vi "Edit_Maths_Equation.vi"(3 "Template Info Array":T1[](array[typedef]) {"Tolerance" min=0.0 format="%#.4f"}, 4 "Maths Equation In":string, 5 "Channel Name":string) -> (0 "Template Info Array Out":T1[](array[typedef]) {"Tolerance" min=0.0 format="%#.4f"}, 1 "Maths Equation Out":string)   [LabVIEW 2016]
uses:
  File_Template_Clus.ctl
  Data plotting/subVIs/Dispose_Channel.ctl
panel:
  in  "K 9":u16(ring) items=["File::", "Date::", "Time::", "Comments::", "Chilled Water:Temp:", "Inlet_Temp:Average:", "Av:Floor:Temp", "Max:deltaT:", "X (mm)::", "Y (mm)::", "Z (mm)::", "Z (m)::", "U/Uref::", "u^2/Uref^2::", "w^2/Uref^2::", "-uw/Uref^2::", "Inlet:DeltaT:", "DeltaT::", "t^2::", "ut::", "wt::", "Grad:Ri:", "Flux:Ri:", "B-V:Freq:N", "DeltaT/DeltaTmax::", "W/Uref::", "T:thermistor:", "dT/dZ::", "dU/dZ::", "Inlet:Delta_Set:", "u'/U::", "w'/U::", "W/U::", "Location:XY:", "Location:XZ:", "U:m/s:", "W:m/s:", "u^2::", "w^2::", "Speed/Uref::", "T:cw:", "Uref::", "Flow:Meas:Time", "Profile::", "t'/T::", "t'::", "uw::", "Spires::", "Roughness::", "Z=1450:Inlet:Temp", "Z=1350:Inlet:Temp", "Z=1250:Inlet:Temp", "Z=1150:Inlet:Temp", "Z=1050:Inlet:Temp", "Z=950:Inlet:Temp", "Z=850:Inlet:Temp", "Z=750:Inlet:Temp", "Z=650:Inlet:Temp", "Z=550:Inlet:Temp", "Z=450:Inlet:Temp", "Z=350:Inlet:Temp", "Z=250:Inlet:Temp", "Z=150:Inlet:Temp", "Z=50:Inlet:Temp", "EnFlo Lab:Hygrometry:Dew Point temp", "EnFlo Lab:Hygrometry:Dew Point temp_PN", "Multi Run:Start Time:", "T cw:Offset:A", "T cw:Grad:B", "LDA (U):Standard Error:in Variance", "LDA (U):Standard Error:in Mean", "LDA (W):Standard Error:in Mean", "LDA (W):Standard Error:in Variance", "U/Uref::Err", "u^2/Uref^2::Err", "W/Uref::Err", "w^2/Uref^2::Err", "Inlet Temp::", "Inlet Setpoint::", "Inlet:Temp:Error", "Seconds:since:1st Jan", "Uni:Chilled Water:Temp", "EnFlo_Tunnel:Chilled Water:Valve Dem Pos", "EnFlo_Tunnel:Temp:Floor_Up_Y=-1585", "EnFlo_Tunnel:Temp:Floor_Up_Y=-1250", "EnFlo_Tunnel:Temp:Floor_Up_Y=-920", "EnFlo_Tunnel:Temp:Floor_Up_Y=-585", "EnFlo_Tunnel:Temp:Floor_Up_Y=-250", "EnFlo_Tunnel:Temp:Floor_Up_Y=80", "EnFlo_Tunnel:Temp:Floor_Up_Y=415", "EnFlo_Tunnel:Temp:Floor_Up_Y=750", "EnFlo_Tunnel:Temp:Floor_Up_Y=1080", "EnFlo_Tunnel:Temp:Floor_Up_Y=1415", "Raw:Data:Filename", "Z=1450:Inlet:Setpoint", "Z=1350:Inlet:Setpoint", "Z=1250:Inlet:Setpoint", "Z=1150:Inlet:Setpoint", "Z=1050:Inlet:Setpoint", "Z=950:Inlet:Setpoint", "Z=850:Inlet:Setpoint", "Z=750:Inlet:Setpoint", "Z=650:Inlet:Setpoint", "Z=550:Inlet:Setpoint", "Z=450:Inlet:Setpoint", "Z=350:Inlet:Setpoint", "Z=250:Inlet:Setpoint", "Z=150:Inlet:Setpoint", "Z=50:Inlet:Setpoint", "Freq:Hz:", "LDA (U):E(f):", "LDA (W):E(f):", "CW (T):f.E(f):", "LDA (U):f.E(f):", "LDA (W):f.E(f):", "Folder::", "Inst::"]
  in  "String 18":string
  in  "K 8":u16(ring) items=["File::", "Date::", "Time::", "Comments::", "Chilled Water:Temp:", "Inlet_Temp:Average:", "Av:Floor:Temp", "Max:deltaT:", "X (mm)::", "Y (mm)::", "Z (mm)::", "Z (m)::", "U/Uref::", "u^2/Uref^2::", "w^2/Uref^2::", "-uw/Uref^2::", "Inlet:DeltaT:", "DeltaT::", "t^2::", "ut::", "wt::", "Grad:Ri:", "Flux:Ri:", "B-V:Freq:N", "DeltaT/DeltaTmax::", "W/Uref::", "T:thermistor:", "dT/dZ::", "dU/dZ::", "Inlet:Delta_Set:", "u'/U::", "w'/U::", "W/U::", "Location:XY:", "Location:XZ:", "U:m/s:", "W:m/s:", "u^2::", "w^2::", "Speed/Uref::", "T:cw:", "Uref::", "Flow:Meas:Time", "Profile::", "t'/T::", "t'::", "uw::", "Spires::", "Roughness::", "Z=1450:Inlet:Temp", "Z=1350:Inlet:Temp", "Z=1250:Inlet:Temp", "Z=1150:Inlet:Temp", "Z=1050:Inlet:Temp", "Z=950:Inlet:Temp", "Z=850:Inlet:Temp", "Z=750:Inlet:Temp", "Z=650:Inlet:Temp", "Z=550:Inlet:Temp", "Z=450:Inlet:Temp", "Z=350:Inlet:Temp", "Z=250:Inlet:Temp", "Z=150:Inlet:Temp", "Z=50:Inlet:Temp", "EnFlo Lab:Hygrometry:Dew Point temp", "EnFlo Lab:Hygrometry:Dew Point temp_PN", "Multi Run:Start Time:", "T cw:Offset:A", "T cw:Grad:B", "LDA (U):Standard Error:in Variance", "LDA (U):Standard Error:in Mean", "LDA (W):Standard Error:in Mean", "LDA (W):Standard Error:in Variance", "U/Uref::Err", "u^2/Uref^2::Err", "W/Uref::Err", "w^2/Uref^2::Err", "Inlet Temp::", "Inlet Setpoint::", "Inlet:Temp:Error", "Seconds:since:1st Jan", "Uni:Chilled Water:Temp", "EnFlo_Tunnel:Chilled Water:Valve Dem Pos", "EnFlo_Tunnel:Temp:Floor_Up_Y=-1585", "EnFlo_Tunnel:Temp:Floor_Up_Y=-1250", "EnFlo_Tunnel:Temp:Floor_Up_Y=-920", "EnFlo_Tunnel:Temp:Floor_Up_Y=-585", "EnFlo_Tunnel:Temp:Floor_Up_Y=-250", "EnFlo_Tunnel:Temp:Floor_Up_Y=80", "EnFlo_Tunnel:Temp:Floor_Up_Y=415", "EnFlo_Tunnel:Temp:Floor_Up_Y=750", "EnFlo_Tunnel:Temp:Floor_Up_Y=1080", "EnFlo_Tunnel:Temp:Floor_Up_Y=1415", "Raw:Data:Filename", "Z=1450:Inlet:Setpoint", "Z=1350:Inlet:Setpoint", "Z=1250:Inlet:Setpoint", "Z=1150:Inlet:Setpoint", "Z=1050:Inlet:Setpoint", "Z=950:Inlet:Setpoint", "Z=850:Inlet:Setpoint", "Z=750:Inlet:Setpoint", "Z=650:Inlet:Setpoint", "Z=550:Inlet:Setpoint", "Z=450:Inlet:Setpoint", "Z=350:Inlet:Setpoint", "Z=250:Inlet:Setpoint", "Z=150:Inlet:Setpoint", "Z=50:Inlet:Setpoint", "Freq:Hz:", "LDA (U):E(f):", "LDA (W):E(f):", "CW (T):f.E(f):", "LDA (U):f.E(f):", "LDA (W):f.E(f):", "Folder::", "Inst::"]
  in  "String 17":string
  in  "K 7":u16(ring) items=["File::", "Date::", "Time::", "Comments::", "Chilled Water:Temp:", "Inlet_Temp:Average:", "Av:Floor:Temp", "Max:deltaT:", "X (mm)::", "Y (mm)::", "Z (mm)::", "Z (m)::", "U/Uref::", "u^2/Uref^2::", "w^2/Uref^2::", "-uw/Uref^2::", "Inlet:DeltaT:", "DeltaT::", "t^2::", "ut::", "wt::", "Grad:Ri:", "Flux:Ri:", "B-V:Freq:N", "DeltaT/DeltaTmax::", "W/Uref::", "T:thermistor:", "dT/dZ::", "dU/dZ::", "Inlet:Delta_Set:", "u'/U::", "w'/U::", "W/U::", "Location:XY:", "Location:XZ:", "U:m/s:", "W:m/s:", "u^2::", "w^2::", "Speed/Uref::", "T:cw:", "Uref::", "Flow:Meas:Time", "Profile::", "t'/T::", "t'::", "uw::", "Spires::", "Roughness::", "Z=1450:Inlet:Temp", "Z=1350:Inlet:Temp", "Z=1250:Inlet:Temp", "Z=1150:Inlet:Temp", "Z=1050:Inlet:Temp", "Z=950:Inlet:Temp", "Z=850:Inlet:Temp", "Z=750:Inlet:Temp", "Z=650:Inlet:Temp", "Z=550:Inlet:Temp", "Z=450:Inlet:Temp", "Z=350:Inlet:Temp", "Z=250:Inlet:Temp", "Z=150:Inlet:Temp", "Z=50:Inlet:Temp", "EnFlo Lab:Hygrometry:Dew Point temp", "EnFlo Lab:Hygrometry:Dew Point temp_PN", "Multi Run:Start Time:", "T cw:Offset:A", "T cw:Grad:B", "LDA (U):Standard Error:in Variance", "LDA (U):Standard Error:in Mean", "LDA (W):Standard Error:in Mean", "LDA (W):Standard Error:in Variance", "U/Uref::Err", "u^2/Uref^2::Err", "W/Uref::Err", "w^2/Uref^2::Err", "Inlet Temp::", "Inlet Setpoint::", "Inlet:Temp:Error", "Seconds:since:1st Jan", "Uni:Chilled Water:Temp", "EnFlo_Tunnel:Chilled Water:Valve Dem Pos", "EnFlo_Tunnel:Temp:Floor_Up_Y=-1585", "EnFlo_Tunnel:Temp:Floor_Up_Y=-1250", "EnFlo_Tunnel:Temp:Floor_Up_Y=-920", "EnFlo_Tunnel:Temp:Floor_Up_Y=-585", "EnFlo_Tunnel:Temp:Floor_Up_Y=-250", "EnFlo_Tunnel:Temp:Floor_Up_Y=80", "EnFlo_Tunnel:Temp:Floor_Up_Y=415", "EnFlo_Tunnel:Temp:Floor_Up_Y=750", "EnFlo_Tunnel:Temp:Floor_Up_Y=1080", "EnFlo_Tunnel:Temp:Floor_Up_Y=1415", "Raw:Data:Filename", "Z=1450:Inlet:Setpoint", "Z=1350:Inlet:Setpoint", "Z=1250:Inlet:Setpoint", "Z=1150:Inlet:Setpoint", "Z=1050:Inlet:Setpoint", "Z=950:Inlet:Setpoint", "Z=850:Inlet:Setpoint", "Z=750:Inlet:Setpoint", "Z=650:Inlet:Setpoint", "Z=550:Inlet:Setpoint", "Z=450:Inlet:Setpoint", "Z=350:Inlet:Setpoint", "Z=250:Inlet:Setpoint", "Z=150:Inlet:Setpoint", "Z=50:Inlet:Setpoint", "Freq:Hz:", "LDA (U):E(f):", "LDA (W):E(f):", "CW (T):f.E(f):", "LDA (U):f.E(f):", "LDA (W):f.E(f):", "Folder::", "Inst::"]
  in  "String 16":string
  in  "K 6":u16(ring) items=["File::", "Date::", "Time::", "Comments::", "Chilled Water:Temp:", "Inlet_Temp:Average:", "Av:Floor:Temp", "Max:deltaT:", "X (mm)::", "Y (mm)::", "Z (mm)::", "Z (m)::", "U/Uref::", "u^2/Uref^2::", "w^2/Uref^2::", "-uw/Uref^2::", "Inlet:DeltaT:", "DeltaT::", "t^2::", "ut::", "wt::", "Grad:Ri:", "Flux:Ri:", "B-V:Freq:N", "DeltaT/DeltaTmax::", "W/Uref::", "T:thermistor:", "dT/dZ::", "dU/dZ::", "Inlet:Delta_Set:", "u'/U::", "w'/U::", "W/U::", "Location:XY:", "Location:XZ:", "U:m/s:", "W:m/s:", "u^2::", "w^2::", "Speed/Uref::", "T:cw:", "Uref::", "Flow:Meas:Time", "Profile::", "t'/T::", "t'::", "uw::", "Spires::", "Roughness::", "Z=1450:Inlet:Temp", "Z=1350:Inlet:Temp", "Z=1250:Inlet:Temp", "Z=1150:Inlet:Temp", "Z=1050:Inlet:Temp", "Z=950:Inlet:Temp", "Z=850:Inlet:Temp", "Z=750:Inlet:Temp", "Z=650:Inlet:Temp", "Z=550:Inlet:Temp", "Z=450:Inlet:Temp", "Z=350:Inlet:Temp", "Z=250:Inlet:Temp", "Z=150:Inlet:Temp", "Z=50:Inlet:Temp", "EnFlo Lab:Hygrometry:Dew Point temp", "EnFlo Lab:Hygrometry:Dew Point temp_PN", "Multi Run:Start Time:", "T cw:Offset:A", "T cw:Grad:B", "LDA (U):Standard Error:in Variance", "LDA (U):Standard Error:in Mean", "LDA (W):Standard Error:in Mean", "LDA (W):Standard Error:in Variance", "U/Uref::Err", "u^2/Uref^2::Err", "W/Uref::Err", "w^2/Uref^2::Err", "Inlet Temp::", "Inlet Setpoint::", "Inlet:Temp:Error", "Seconds:since:1st Jan", "Uni:Chilled Water:Temp", "EnFlo_Tunnel:Chilled Water:Valve Dem Pos", "EnFlo_Tunnel:Temp:Floor_Up_Y=-1585", "EnFlo_Tunnel:Temp:Floor_Up_Y=-1250", "EnFlo_Tunnel:Temp:Floor_Up_Y=-920", "EnFlo_Tunnel:Temp:Floor_Up_Y=-585", "EnFlo_Tunnel:Temp:Floor_Up_Y=-250", "EnFlo_Tunnel:Temp:Floor_Up_Y=80", "EnFlo_Tunnel:Temp:Floor_Up_Y=415", "EnFlo_Tunnel:Temp:Floor_Up_Y=750", "EnFlo_Tunnel:Temp:Floor_Up_Y=1080", "EnFlo_Tunnel:Temp:Floor_Up_Y=1415", "Raw:Data:Filename", "Z=1450:Inlet:Setpoint", "Z=1350:Inlet:Setpoint", "Z=1250:Inlet:Setpoint", "Z=1150:Inlet:Setpoint", "Z=1050:Inlet:Setpoint", "Z=950:Inlet:Setpoint", "Z=850:Inlet:Setpoint", "Z=750:Inlet:Setpoint", "Z=650:Inlet:Setpoint", "Z=550:Inlet:Setpoint", "Z=450:Inlet:Setpoint", "Z=350:Inlet:Setpoint", "Z=250:Inlet:Setpoint", "Z=150:Inlet:Setpoint", "Z=50:Inlet:Setpoint", "Freq:Hz:", "LDA (U):E(f):", "LDA (W):E(f):", "CW (T):f.E(f):", "LDA (U):f.E(f):", "LDA (W):f.E(f):", "Folder::", "Inst::"]
  in  "String 15":string
  in  "K 5":u16(ring) items=["File::", "Date::", "Time::", "Comments::", "Chilled Water:Temp:", "Inlet_Temp:Average:", "Av:Floor:Temp", "Max:deltaT:", "X (mm)::", "Y (mm)::", "Z (mm)::", "Z (m)::", "U/Uref::", "u^2/Uref^2::", "w^2/Uref^2::", "-uw/Uref^2::", "Inlet:DeltaT:", "DeltaT::", "t^2::", "ut::", "wt::", "Grad:Ri:", "Flux:Ri:", "B-V:Freq:N", "DeltaT/DeltaTmax::", "W/Uref::", "T:thermistor:", "dT/dZ::", "dU/dZ::", "Inlet:Delta_Set:", "u'/U::", "w'/U::", "W/U::", "Location:XY:", "Location:XZ:", "U:m/s:", "W:m/s:", "u^2::", "w^2::", "Speed/Uref::", "T:cw:", "Uref::", "Flow:Meas:Time", "Profile::", "t'/T::", "t'::", "uw::", "Spires::", "Roughness::", "Z=1450:Inlet:Temp", "Z=1350:Inlet:Temp", "Z=1250:Inlet:Temp", "Z=1150:Inlet:Temp", "Z=1050:Inlet:Temp", "Z=950:Inlet:Temp", "Z=850:Inlet:Temp", "Z=750:Inlet:Temp", "Z=650:Inlet:Temp", "Z=550:Inlet:Temp", "Z=450:Inlet:Temp", "Z=350:Inlet:Temp", "Z=250:Inlet:Temp", "Z=150:Inlet:Temp", "Z=50:Inlet:Temp", "EnFlo Lab:Hygrometry:Dew Point temp", "EnFlo Lab:Hygrometry:Dew Point temp_PN", "Multi Run:Start Time:", "T cw:Offset:A", "T cw:Grad:B", "LDA (U):Standard Error:in Variance", "LDA (U):Standard Error:in Mean", "LDA (W):Standard Error:in Mean", "LDA (W):Standard Error:in Variance", "U/Uref::Err", "u^2/Uref^2::Err", "W/Uref::Err", "w^2/Uref^2::Err", "Inlet Temp::", "Inlet Setpoint::", "Inlet:Temp:Error", "Seconds:since:1st Jan", "Uni:Chilled Water:Temp", "EnFlo_Tunnel:Chilled Water:Valve Dem Pos", "EnFlo_Tunnel:Temp:Floor_Up_Y=-1585", "EnFlo_Tunnel:Temp:Floor_Up_Y=-1250", "EnFlo_Tunnel:Temp:Floor_Up_Y=-920", "EnFlo_Tunnel:Temp:Floor_Up_Y=-585", "EnFlo_Tunnel:Temp:Floor_Up_Y=-250", "EnFlo_Tunnel:Temp:Floor_Up_Y=80", "EnFlo_Tunnel:Temp:Floor_Up_Y=415", "EnFlo_Tunnel:Temp:Floor_Up_Y=750", "EnFlo_Tunnel:Temp:Floor_Up_Y=1080", "EnFlo_Tunnel:Temp:Floor_Up_Y=1415", "Raw:Data:Filename", "Z=1450:Inlet:Setpoint", "Z=1350:Inlet:Setpoint", "Z=1250:Inlet:Setpoint", "Z=1150:Inlet:Setpoint", "Z=1050:Inlet:Setpoint", "Z=950:Inlet:Setpoint", "Z=850:Inlet:Setpoint", "Z=750:Inlet:Setpoint", "Z=650:Inlet:Setpoint", "Z=550:Inlet:Setpoint", "Z=450:Inlet:Setpoint", "Z=350:Inlet:Setpoint", "Z=250:Inlet:Setpoint", "Z=150:Inlet:Setpoint", "Z=50:Inlet:Setpoint", "Freq:Hz:", "LDA (U):E(f):", "LDA (W):E(f):", "CW (T):f.E(f):", "LDA (U):f.E(f):", "LDA (W):f.E(f):", "Folder::", "Inst::"]
  in  "String 14":string
  in  "N":u16(ring) items=["File::", "Date::", "Time::", "Comments::", "Chilled Water:Temp:", "Inlet_Temp:Average:", "Av:Floor:Temp", "Max:deltaT:", "X (mm)::", "Y (mm)::", "Z (mm)::", "Z (m)::", "U/Uref::", "u^2/Uref^2::", "w^2/Uref^2::", "-uw/Uref^2::", "Inlet:DeltaT:", "DeltaT::", "t^2::", "ut::", "wt::", "Grad:Ri:", "Flux:Ri:", "B-V:Freq:N", "DeltaT/DeltaTmax::", "W/Uref::", "T:thermistor:", "dT/dZ::", "dU/dZ::", "Inlet:Delta_Set:", "u'/U::", "w'/U::", "W/U::", "Location:XY:", "Location:XZ:", "U:m/s:", "W:m/s:", "u^2::", "w^2::", "Speed/Uref::", "T:cw:", "Uref::", "Flow:Meas:Time", "Profile::", "t'/T::", "t'::", "uw::", "Spires::", "Roughness::", "Z=1450:Inlet:Temp", "Z=1350:Inlet:Temp", "Z=1250:Inlet:Temp", "Z=1150:Inlet:Temp", "Z=1050:Inlet:Temp", "Z=950:Inlet:Temp", "Z=850:Inlet:Temp", "Z=750:Inlet:Temp", "Z=650:Inlet:Temp", "Z=550:Inlet:Temp", "Z=450:Inlet:Temp", "Z=350:Inlet:Temp", "Z=250:Inlet:Temp", "Z=150:Inlet:Temp", "Z=50:Inlet:Temp", "EnFlo Lab:Hygrometry:Dew Point temp", "EnFlo Lab:Hygrometry:Dew Point temp_PN", "Multi Run:Start Time:", "T cw:Offset:A", "T cw:Grad:B", "LDA (U):Standard Error:in Variance", "LDA (U):Standard Error:in Mean", "LDA (W):Standard Error:in Mean", "LDA (W):Standard Error:in Variance", "U/Uref::Err", "u^2/Uref^2::Err", "W/Uref::Err", "w^2/Uref^2::Err", "Inlet Temp::", "Inlet Setpoint::", "Inlet:Temp:Error", "Seconds:since:1st Jan", "Uni:Chilled Water:Temp", "EnFlo_Tunnel:Chilled Water:Valve Dem Pos", "EnFlo_Tunnel:Temp:Floor_Up_Y=-1585", "EnFlo_Tunnel:Temp:Floor_Up_Y=-1250", "EnFlo_Tunnel:Temp:Floor_Up_Y=-920", "EnFlo_Tunnel:Temp:Floor_Up_Y=-585", "EnFlo_Tunnel:Temp:Floor_Up_Y=-250", "EnFlo_Tunnel:Temp:Floor_Up_Y=80", "EnFlo_Tunnel:Temp:Floor_Up_Y=415", "EnFlo_Tunnel:Temp:Floor_Up_Y=750", "EnFlo_Tunnel:Temp:Floor_Up_Y=1080", "EnFlo_Tunnel:Temp:Floor_Up_Y=1415", "Raw:Data:Filename", "Z=1450:Inlet:Setpoint", "Z=1350:Inlet:Setpoint", "Z=1250:Inlet:Setpoint", "Z=1150:Inlet:Setpoint", "Z=1050:Inlet:Setpoint", "Z=950:Inlet:Setpoint", "Z=850:Inlet:Setpoint", "Z=750:Inlet:Setpoint", "Z=650:Inlet:Setpoint", "Z=550:Inlet:Setpoint", "Z=450:Inlet:Setpoint", "Z=350:Inlet:Setpoint", "Z=250:Inlet:Setpoint", "Z=150:Inlet:Setpoint", "Z=50:Inlet:Setpoint", "Freq:Hz:", "LDA (U):E(f):", "LDA (W):E(f):", "CW (T):f.E(f):", "LDA (U):f.E(f):", "LDA (W):f.E(f):", "Folder::", "Inst::"]
  in  "String 13":string
  in  "M":u16(ring) items=["File::", "Date::", "Time::", "Comments::", "Chilled Water:Temp:", "Inlet_Temp:Average:", "Av:Floor:Temp", "Max:deltaT:", "X (mm)::", "Y (mm)::", "Z (mm)::", "Z (m)::", "U/Uref::", "u^2/Uref^2::", "w^2/Uref^2::", "-uw/Uref^2::", "Inlet:DeltaT:", "DeltaT::", "t^2::", "ut::", "wt::", "Grad:Ri:", "Flux:Ri:", "B-V:Freq:N", "DeltaT/DeltaTmax::", "W/Uref::", "T:thermistor:", "dT/dZ::", "dU/dZ::", "Inlet:Delta_Set:", "u'/U::", "w'/U::", "W/U::", "Location:XY:", "Location:XZ:", "U:m/s:", "W:m/s:", "u^2::", "w^2::", "Speed/Uref::", "T:cw:", "Uref::", "Flow:Meas:Time", "Profile::", "t'/T::", "t'::", "uw::", "Spires::", "Roughness::", "Z=1450:Inlet:Temp", "Z=1350:Inlet:Temp", "Z=1250:Inlet:Temp", "Z=1150:Inlet:Temp", "Z=1050:Inlet:Temp", "Z=950:Inlet:Temp", "Z=850:Inlet:Temp", "Z=750:Inlet:Temp", "Z=650:Inlet:Temp", "Z=550:Inlet:Temp", "Z=450:Inlet:Temp", "Z=350:Inlet:Temp", "Z=250:Inlet:Temp", "Z=150:Inlet:Temp", "Z=50:Inlet:Temp", "EnFlo Lab:Hygrometry:Dew Point temp", "EnFlo Lab:Hygrometry:Dew Point temp_PN", "Multi Run:Start Time:", "T cw:Offset:A", "T cw:Grad:B", "LDA (U):Standard Error:in Variance", "LDA (U):Standard Error:in Mean", "LDA (W):Standard Error:in Mean", "LDA (W):Standard Error:in Variance", "U/Uref::Err", "u^2/Uref^2::Err", "W/Uref::Err", "w^2/Uref^2::Err", "Inlet Temp::", "Inlet Setpoint::", "Inlet:Temp:Error", "Seconds:since:1st Jan", "Uni:Chilled Water:Temp", "EnFlo_Tunnel:Chilled Water:Valve Dem Pos", "EnFlo_Tunnel:Temp:Floor_Up_Y=-1585", "EnFlo_Tunnel:Temp:Floor_Up_Y=-1250", "EnFlo_Tunnel:Temp:Floor_Up_Y=-920", "EnFlo_Tunnel:Temp:Floor_Up_Y=-585", "EnFlo_Tunnel:Temp:Floor_Up_Y=-250", "EnFlo_Tunnel:Temp:Floor_Up_Y=80", "EnFlo_Tunnel:Temp:Floor_Up_Y=415", "EnFlo_Tunnel:Temp:Floor_Up_Y=750", "EnFlo_Tunnel:Temp:Floor_Up_Y=1080", "EnFlo_Tunnel:Temp:Floor_Up_Y=1415", "Raw:Data:Filename", "Z=1450:Inlet:Setpoint", "Z=1350:Inlet:Setpoint", "Z=1250:Inlet:Setpoint", "Z=1150:Inlet:Setpoint", "Z=1050:Inlet:Setpoint", "Z=950:Inlet:Setpoint", "Z=850:Inlet:Setpoint", "Z=750:Inlet:Setpoint", "Z=650:Inlet:Setpoint", "Z=550:Inlet:Setpoint", "Z=450:Inlet:Setpoint", "Z=350:Inlet:Setpoint", "Z=250:Inlet:Setpoint", "Z=150:Inlet:Setpoint", "Z=50:Inlet:Setpoint", "Freq:Hz:", "LDA (U):E(f):", "LDA (W):E(f):", "CW (T):f.E(f):", "LDA (U):f.E(f):", "LDA (W):f.E(f):", "Folder::", "Inst::"]
  in  "String 12":string
  in  "L":u16(ring) items=["File::", "Date::", "Time::", "Comments::", "Chilled Water:Temp:", "Inlet_Temp:Average:", "Av:Floor:Temp", "Max:deltaT:", "X (mm)::", "Y (mm)::", "Z (mm)::", "Z (m)::", "U/Uref::", "u^2/Uref^2::", "w^2/Uref^2::", "-uw/Uref^2::", "Inlet:DeltaT:", "DeltaT::", "t^2::", "ut::", "wt::", "Grad:Ri:", "Flux:Ri:", "B-V:Freq:N", "DeltaT/DeltaTmax::", "W/Uref::", "T:thermistor:", "dT/dZ::", "dU/dZ::", "Inlet:Delta_Set:", "u'/U::", "w'/U::", "W/U::", "Location:XY:", "Location:XZ:", "U:m/s:", "W:m/s:", "u^2::", "w^2::", "Speed/Uref::", "T:cw:", "Uref::", "Flow:Meas:Time", "Profile::", "t'/T::", "t'::", "uw::", "Spires::", "Roughness::", "Z=1450:Inlet:Temp", "Z=1350:Inlet:Temp", "Z=1250:Inlet:Temp", "Z=1150:Inlet:Temp", "Z=1050:Inlet:Temp", "Z=950:Inlet:Temp", "Z=850:Inlet:Temp", "Z=750:Inlet:Temp", "Z=650:Inlet:Temp", "Z=550:Inlet:Temp", "Z=450:Inlet:Temp", "Z=350:Inlet:Temp", "Z=250:Inlet:Temp", "Z=150:Inlet:Temp", "Z=50:Inlet:Temp", "EnFlo Lab:Hygrometry:Dew Point temp", "EnFlo Lab:Hygrometry:Dew Point temp_PN", "Multi Run:Start Time:", "T cw:Offset:A", "T cw:Grad:B", "LDA (U):Standard Error:in Variance", "LDA (U):Standard Error:in Mean", "LDA (W):Standard Error:in Mean", "LDA (W):Standard Error:in Variance", "U/Uref::Err", "u^2/Uref^2::Err", "W/Uref::Err", "w^2/Uref^2::Err", "Inlet Temp::", "Inlet Setpoint::", "Inlet:Temp:Error", "Seconds:since:1st Jan", "Uni:Chilled Water:Temp", "EnFlo_Tunnel:Chilled Water:Valve Dem Pos", "EnFlo_Tunnel:Temp:Floor_Up_Y=-1585", "EnFlo_Tunnel:Temp:Floor_Up_Y=-1250", "EnFlo_Tunnel:Temp:Floor_Up_Y=-920", "EnFlo_Tunnel:Temp:Floor_Up_Y=-585", "EnFlo_Tunnel:Temp:Floor_Up_Y=-250", "EnFlo_Tunnel:Temp:Floor_Up_Y=80", "EnFlo_Tunnel:Temp:Floor_Up_Y=415", "EnFlo_Tunnel:Temp:Floor_Up_Y=750", "EnFlo_Tunnel:Temp:Floor_Up_Y=1080", "EnFlo_Tunnel:Temp:Floor_Up_Y=1415", "Raw:Data:Filename", "Z=1450:Inlet:Setpoint", "Z=1350:Inlet:Setpoint", "Z=1250:Inlet:Setpoint", "Z=1150:Inlet:Setpoint", "Z=1050:Inlet:Setpoint", "Z=950:Inlet:Setpoint", "Z=850:Inlet:Setpoint", "Z=750:Inlet:Setpoint", "Z=650:Inlet:Setpoint", "Z=550:Inlet:Setpoint", "Z=450:Inlet:Setpoint", "Z=350:Inlet:Setpoint", "Z=250:Inlet:Setpoint", "Z=150:Inlet:Setpoint", "Z=50:Inlet:Setpoint", "Freq:Hz:", "LDA (U):E(f):", "LDA (W):E(f):", "CW (T):f.E(f):", "LDA (U):f.E(f):", "LDA (W):f.E(f):", "Folder::", "Inst::"]
  in  "String 11":string
  out "Maths Equation Symbols":string
  in  "Start String":string
  in  "K":u16(ring) items=["File::", "Date::", "Time::", "Comments::", "Chilled Water:Temp:", "Inlet_Temp:Average:", "Av:Floor:Temp", "Max:deltaT:", "X (mm)::", "Y (mm)::", "Z (mm)::", "Z (m)::", "U/Uref::", "u^2/Uref^2::", "w^2/Uref^2::", "-uw/Uref^2::", "Inlet:DeltaT:", "DeltaT::", "t^2::", "ut::", "wt::", "Grad:Ri:", "Flux:Ri:", "B-V:Freq:N", "DeltaT/DeltaTmax::", "W/Uref::", "T:thermistor:", "dT/dZ::", "dU/dZ::", "Inlet:Delta_Set:", "u'/U::", "w'/U::", "W/U::", "Location:XY:", "Location:XZ:", "U:m/s:", "W:m/s:", "u^2::", "w^2::", "Speed/Uref::", "T:cw:", "Uref::", "Flow:Meas:Time", "Profile::", "t'/T::", "t'::", "uw::", "Spires::", "Roughness::", "Z=1450:Inlet:Temp", "Z=1350:Inlet:Temp", "Z=1250:Inlet:Temp", "Z=1150:Inlet:Temp", "Z=1050:Inlet:Temp", "Z=950:Inlet:Temp", "Z=850:Inlet:Temp", "Z=750:Inlet:Temp", "Z=650:Inlet:Temp", "Z=550:Inlet:Temp", "Z=450:Inlet:Temp", "Z=350:Inlet:Temp", "Z=250:Inlet:Temp", "Z=150:Inlet:Temp", "Z=50:Inlet:Temp", "EnFlo Lab:Hygrometry:Dew Point temp", "EnFlo Lab:Hygrometry:Dew Point temp_PN", "Multi Run:Start Time:", "T cw:Offset:A", "T cw:Grad:B", "LDA (U):Standard Error:in Variance", "LDA (U):Standard Error:in Mean", "LDA (W):Standard Error:in Mean", "LDA (W):Standard Error:in Variance", "U/Uref::Err", "u^2/Uref^2::Err", "W/Uref::Err", "w^2/Uref^2::Err", "Inlet Temp::", "Inlet Setpoint::", "Inlet:Temp:Error", "Seconds:since:1st Jan", "Uni:Chilled Water:Temp", "EnFlo_Tunnel:Chilled Water:Valve Dem Pos", "EnFlo_Tunnel:Temp:Floor_Up_Y=-1585", "EnFlo_Tunnel:Temp:Floor_Up_Y=-1250", "EnFlo_Tunnel:Temp:Floor_Up_Y=-920", "EnFlo_Tunnel:Temp:Floor_Up_Y=-585", "EnFlo_Tunnel:Temp:Floor_Up_Y=-250", "EnFlo_Tunnel:Temp:Floor_Up_Y=80", "EnFlo_Tunnel:Temp:Floor_Up_Y=415", "EnFlo_Tunnel:Temp:Floor_Up_Y=750", "EnFlo_Tunnel:Temp:Floor_Up_Y=1080", "EnFlo_Tunnel:Temp:Floor_Up_Y=1415", "Raw:Data:Filename", "Z=1450:Inlet:Setpoint", "Z=1350:Inlet:Setpoint", "Z=1250:Inlet:Setpoint", "Z=1150:Inlet:Setpoint", "Z=1050:Inlet:Setpoint", "Z=950:Inlet:Setpoint", "Z=850:Inlet:Setpoint", "Z=750:Inlet:Setpoint", "Z=650:Inlet:Setpoint", "Z=550:Inlet:Setpoint", "Z=450:Inlet:Setpoint", "Z=350:Inlet:Setpoint", "Z=250:Inlet:Setpoint", "Z=150:Inlet:Setpoint", "Z=50:Inlet:Setpoint", "Freq:Hz:", "LDA (U):E(f):", "LDA (W):E(f):", "CW (T):f.E(f):", "LDA (U):f.E(f):", "LDA (W):f.E(f):", "Folder::", "Inst::"]
  in  "String 10":string
  in  "J":u16(ring) items=["File::", "Date::", "Time::", "Comments::", "Chilled Water:Temp:", "Inlet_Temp:Average:", "Av:Floor:Temp", "Max:deltaT:", "X (mm)::", "Y (mm)::", "Z (mm)::", "Z (m)::", "U/Uref::", "u^2/Uref^2::", "w^2/Uref^2::", "-uw/Uref^2::", "Inlet:DeltaT:", "DeltaT::", "t^2::", "ut::", "wt::", "Grad:Ri:", "Flux:Ri:", "B-V:Freq:N", "DeltaT/DeltaTmax::", "W/Uref::", "T:thermistor:", "dT/dZ::", "dU/dZ::", "Inlet:Delta_Set:", "u'/U::", "w'/U::", "W/U::", "Location:XY:", "Location:XZ:", "U:m/s:", "W:m/s:", "u^2::", "w^2::", "Speed/Uref::", "T:cw:", "Uref::", "Flow:Meas:Time", "Profile::", "t'/T::", "t'::", "uw::", "Spires::", "Roughness::", "Z=1450:Inlet:Temp", "Z=1350:Inlet:Temp", "Z=1250:Inlet:Temp", "Z=1150:Inlet:Temp", "Z=1050:Inlet:Temp", "Z=950:Inlet:Temp", "Z=850:Inlet:Temp", "Z=750:Inlet:Temp", "Z=650:Inlet:Temp", "Z=550:Inlet:Temp", "Z=450:Inlet:Temp", "Z=350:Inlet:Temp", "Z=250:Inlet:Temp", "Z=150:Inlet:Temp", "Z=50:Inlet:Temp", "EnFlo Lab:Hygrometry:Dew Point temp", "EnFlo Lab:Hygrometry:Dew Point temp_PN", "Multi Run:Start Time:", "T cw:Offset:A", "T cw:Grad:B", "LDA (U):Standard Error:in Variance", "LDA (U):Standard Error:in Mean", "LDA (W):Standard Error:in Mean", "LDA (W):Standard Error:in Variance", "U/Uref::Err", "u^2/Uref^2::Err", "W/Uref::Err", "w^2/Uref^2::Err", "Inlet Temp::", "Inlet Setpoint::", "Inlet:Temp:Error", "Seconds:since:1st Jan", "Uni:Chilled Water:Temp", "EnFlo_Tunnel:Chilled Water:Valve Dem Pos", "EnFlo_Tunnel:Temp:Floor_Up_Y=-1585", "EnFlo_Tunnel:Temp:Floor_Up_Y=-1250", "EnFlo_Tunnel:Temp:Floor_Up_Y=-920", "EnFlo_Tunnel:Temp:Floor_Up_Y=-585", "EnFlo_Tunnel:Temp:Floor_Up_Y=-250", "EnFlo_Tunnel:Temp:Floor_Up_Y=80", "EnFlo_Tunnel:Temp:Floor_Up_Y=415", "EnFlo_Tunnel:Temp:Floor_Up_Y=750", "EnFlo_Tunnel:Temp:Floor_Up_Y=1080", "EnFlo_Tunnel:Temp:Floor_Up_Y=1415", "Raw:Data:Filename", "Z=1450:Inlet:Setpoint", "Z=1350:Inlet:Setpoint", "Z=1250:Inlet:Setpoint", "Z=1150:Inlet:Setpoint", "Z=1050:Inlet:Setpoint", "Z=950:Inlet:Setpoint", "Z=850:Inlet:Setpoint", "Z=750:Inlet:Setpoint", "Z=650:Inlet:Setpoint", "Z=550:Inlet:Setpoint", "Z=450:Inlet:Setpoint", "Z=350:Inlet:Setpoint", "Z=250:Inlet:Setpoint", "Z=150:Inlet:Setpoint", "Z=50:Inlet:Setpoint", "Freq:Hz:", "LDA (U):E(f):", "LDA (W):E(f):", "CW (T):f.E(f):", "LDA (U):f.E(f):", "LDA (W):f.E(f):", "Folder::", "Inst::"]
  in  "String 9":string
  in  "H":u16(ring) items=["File::", "Date::", "Time::", "Comments::", "Chilled Water:Temp:", "Inlet_Temp:Average:", "Av:Floor:Temp", "Max:deltaT:", "X (mm)::", "Y (mm)::", "Z (mm)::", "Z (m)::", "U/Uref::", "u^2/Uref^2::", "w^2/Uref^2::", "-uw/Uref^2::", "Inlet:DeltaT:", "DeltaT::", "t^2::", "ut::", "wt::", "Grad:Ri:", "Flux:Ri:", "B-V:Freq:N", "DeltaT/DeltaTmax::", "W/Uref::", "T:thermistor:", "dT/dZ::", "dU/dZ::", "Inlet:Delta_Set:", "u'/U::", "w'/U::", "W/U::", "Location:XY:", "Location:XZ:", "U:m/s:", "W:m/s:", "u^2::", "w^2::", "Speed/Uref::", "T:cw:", "Uref::", "Flow:Meas:Time", "Profile::", "t'/T::", "t'::", "uw::", "Spires::", "Roughness::", "Z=1450:Inlet:Temp", "Z=1350:Inlet:Temp", "Z=1250:Inlet:Temp", "Z=1150:Inlet:Temp", "Z=1050:Inlet:Temp", "Z=950:Inlet:Temp", "Z=850:Inlet:Temp", "Z=750:Inlet:Temp", "Z=650:Inlet:Temp", "Z=550:Inlet:Temp", "Z=450:Inlet:Temp", "Z=350:Inlet:Temp", "Z=250:Inlet:Temp", "Z=150:Inlet:Temp", "Z=50:Inlet:Temp", "EnFlo Lab:Hygrometry:Dew Point temp", "EnFlo Lab:Hygrometry:Dew Point temp_PN", "Multi Run:Start Time:", "T cw:Offset:A", "T cw:Grad:B", "LDA (U):Standard Error:in Variance", "LDA (U):Standard Error:in Mean", "LDA (W):Standard Error:in Mean", "LDA (W):Standard Error:in Variance", "U/Uref::Err", "u^2/Uref^2::Err", "W/Uref::Err", "w^2/Uref^2::Err", "Inlet Temp::", "Inlet Setpoint::", "Inlet:Temp:Error", "Seconds:since:1st Jan", "Uni:Chilled Water:Temp", "EnFlo_Tunnel:Chilled Water:Valve Dem Pos", "EnFlo_Tunnel:Temp:Floor_Up_Y=-1585", "EnFlo_Tunnel:Temp:Floor_Up_Y=-1250", "EnFlo_Tunnel:Temp:Floor_Up_Y=-920", "EnFlo_Tunnel:Temp:Floor_Up_Y=-585", "EnFlo_Tunnel:Temp:Floor_Up_Y=-250", "EnFlo_Tunnel:Temp:Floor_Up_Y=80", "EnFlo_Tunnel:Temp:Floor_Up_Y=415", "EnFlo_Tunnel:Temp:Floor_Up_Y=750", "EnFlo_Tunnel:Temp:Floor_Up_Y=1080", "EnFlo_Tunnel:Temp:Floor_Up_Y=1415", "Raw:Data:Filename", "Z=1450:Inlet:Setpoint", "Z=1350:Inlet:Setpoint", "Z=1250:Inlet:Setpoint", "Z=1150:Inlet:Setpoint", "Z=1050:Inlet:Setpoint", "Z=950:Inlet:Setpoint", "Z=850:Inlet:Setpoint", "Z=750:Inlet:Setpoint", "Z=650:Inlet:Setpoint", "Z=550:Inlet:Setpoint", "Z=450:Inlet:Setpoint", "Z=350:Inlet:Setpoint", "Z=250:Inlet:Setpoint", "Z=150:Inlet:Setpoint", "Z=50:Inlet:Setpoint", "Freq:Hz:", "LDA (U):E(f):", "LDA (W):E(f):", "CW (T):f.E(f):", "LDA (U):f.E(f):", "LDA (W):f.E(f):", "Folder::", "Inst::"]
  in  "String 8":string
  in  "G":u16(ring) items=["File::", "Date::", "Time::", "Comments::", "Chilled Water:Temp:", "Inlet_Temp:Average:", "Av:Floor:Temp", "Max:deltaT:", "X (mm)::", "Y (mm)::", "Z (mm)::", "Z (m)::", "U/Uref::", "u^2/Uref^2::", "w^2/Uref^2::", "-uw/Uref^2::", "Inlet:DeltaT:", "DeltaT::", "t^2::", "ut::", "wt::", "Grad:Ri:", "Flux:Ri:", "B-V:Freq:N", "DeltaT/DeltaTmax::", "W/Uref::", "T:thermistor:", "dT/dZ::", "dU/dZ::", "Inlet:Delta_Set:", "u'/U::", "w'/U::", "W/U::", "Location:XY:", "Location:XZ:", "U:m/s:", "W:m/s:", "u^2::", "w^2::", "Speed/Uref::", "T:cw:", "Uref::", "Flow:Meas:Time", "Profile::", "t'/T::", "t'::", "uw::", "Spires::", "Roughness::", "Z=1450:Inlet:Temp", "Z=1350:Inlet:Temp", "Z=1250:Inlet:Temp", "Z=1150:Inlet:Temp", "Z=1050:Inlet:Temp", "Z=950:Inlet:Temp", "Z=850:Inlet:Temp", "Z=750:Inlet:Temp", "Z=650:Inlet:Temp", "Z=550:Inlet:Temp", "Z=450:Inlet:Temp", "Z=350:Inlet:Temp", "Z=250:Inlet:Temp", "Z=150:Inlet:Temp", "Z=50:Inlet:Temp", "EnFlo Lab:Hygrometry:Dew Point temp", "EnFlo Lab:Hygrometry:Dew Point temp_PN", "Multi Run:Start Time:", "T cw:Offset:A", "T cw:Grad:B", "LDA (U):Standard Error:in Variance", "LDA (U):Standard Error:in Mean", "LDA (W):Standard Error:in Mean", "LDA (W):Standard Error:in Variance", "U/Uref::Err", "u^2/Uref^2::Err", "W/Uref::Err", "w^2/Uref^2::Err", "Inlet Temp::", "Inlet Setpoint::", "Inlet:Temp:Error", "Seconds:since:1st Jan", "Uni:Chilled Water:Temp", "EnFlo_Tunnel:Chilled Water:Valve Dem Pos", "EnFlo_Tunnel:Temp:Floor_Up_Y=-1585", "EnFlo_Tunnel:Temp:Floor_Up_Y=-1250", "EnFlo_Tunnel:Temp:Floor_Up_Y=-920", "EnFlo_Tunnel:Temp:Floor_Up_Y=-585", "EnFlo_Tunnel:Temp:Floor_Up_Y=-250", "EnFlo_Tunnel:Temp:Floor_Up_Y=80", "EnFlo_Tunnel:Temp:Floor_Up_Y=415", "EnFlo_Tunnel:Temp:Floor_Up_Y=750", "EnFlo_Tunnel:Temp:Floor_Up_Y=1080", "EnFlo_Tunnel:Temp:Floor_Up_Y=1415", "Raw:Data:Filename", "Z=1450:Inlet:Setpoint", "Z=1350:Inlet:Setpoint", "Z=1250:Inlet:Setpoint", "Z=1150:Inlet:Setpoint", "Z=1050:Inlet:Setpoint", "Z=950:Inlet:Setpoint", "Z=850:Inlet:Setpoint", "Z=750:Inlet:Setpoint", "Z=650:Inlet:Setpoint", "Z=550:Inlet:Setpoint", "Z=450:Inlet:Setpoint", "Z=350:Inlet:Setpoint", "Z=250:Inlet:Setpoint", "Z=150:Inlet:Setpoint", "Z=50:Inlet:Setpoint", "Freq:Hz:", "LDA (U):E(f):", "LDA (W):E(f):", "CW (T):f.E(f):", "LDA (U):f.E(f):", "LDA (W):f.E(f):", "Folder::", "Inst::"]
  in  "String 7":string
  in  "F":u16(ring) items=["File::", "Date::", "Time::", "Comments::", "Chilled Water:Temp:", "Inlet_Temp:Average:", "Av:Floor:Temp", "Max:deltaT:", "X (mm)::", "Y (mm)::", "Z (mm)::", "Z (m)::", "U/Uref::", "u^2/Uref^2::", "w^2/Uref^2::", "-uw/Uref^2::", "Inlet:DeltaT:", "DeltaT::", "t^2::", "ut::", "wt::", "Grad:Ri:", "Flux:Ri:", "B-V:Freq:N", "DeltaT/DeltaTmax::", "W/Uref::", "T:thermistor:", "dT/dZ::", "dU/dZ::", "Inlet:Delta_Set:", "u'/U::", "w'/U::", "W/U::", "Location:XY:", "Location:XZ:", "U:m/s:", "W:m/s:", "u^2::", "w^2::", "Speed/Uref::", "T:cw:", "Uref::", "Flow:Meas:Time", "Profile::", "t'/T::", "t'::", "uw::", "Spires::", "Roughness::", "Z=1450:Inlet:Temp", "Z=1350:Inlet:Temp", "Z=1250:Inlet:Temp", "Z=1150:Inlet:Temp", "Z=1050:Inlet:Temp", "Z=950:Inlet:Temp", "Z=850:Inlet:Temp", "Z=750:Inlet:Temp", "Z=650:Inlet:Temp", "Z=550:Inlet:Temp", "Z=450:Inlet:Temp", "Z=350:Inlet:Temp", "Z=250:Inlet:Temp", "Z=150:Inlet:Temp", "Z=50:Inlet:Temp", "EnFlo Lab:Hygrometry:Dew Point temp", "EnFlo Lab:Hygrometry:Dew Point temp_PN", "Multi Run:Start Time:", "T cw:Offset:A", "T cw:Grad:B", "LDA (U):Standard Error:in Variance", "LDA (U):Standard Error:in Mean", "LDA (W):Standard Error:in Mean", "LDA (W):Standard Error:in Variance", "U/Uref::Err", "u^2/Uref^2::Err", "W/Uref::Err", "w^2/Uref^2::Err", "Inlet Temp::", "Inlet Setpoint::", "Inlet:Temp:Error", "Seconds:since:1st Jan", "Uni:Chilled Water:Temp", "EnFlo_Tunnel:Chilled Water:Valve Dem Pos", "EnFlo_Tunnel:Temp:Floor_Up_Y=-1585", "EnFlo_Tunnel:Temp:Floor_Up_Y=-1250", "EnFlo_Tunnel:Temp:Floor_Up_Y=-920", "EnFlo_Tunnel:Temp:Floor_Up_Y=-585", "EnFlo_Tunnel:Temp:Floor_Up_Y=-250", "EnFlo_Tunnel:Temp:Floor_Up_Y=80", "EnFlo_Tunnel:Temp:Floor_Up_Y=415", "EnFlo_Tunnel:Temp:Floor_Up_Y=750", "EnFlo_Tunnel:Temp:Floor_Up_Y=1080", "EnFlo_Tunnel:Temp:Floor_Up_Y=1415", "Raw:Data:Filename", "Z=1450:Inlet:Setpoint", "Z=1350:Inlet:Setpoint", "Z=1250:Inlet:Setpoint", "Z=1150:Inlet:Setpoint", "Z=1050:Inlet:Setpoint", "Z=950:Inlet:Setpoint", "Z=850:Inlet:Setpoint", "Z=750:Inlet:Setpoint", "Z=650:Inlet:Setpoint", "Z=550:Inlet:Setpoint", "Z=450:Inlet:Setpoint", "Z=350:Inlet:Setpoint", "Z=250:Inlet:Setpoint", "Z=150:Inlet:Setpoint", "Z=50:Inlet:Setpoint", "Freq:Hz:", "LDA (U):E(f):", "LDA (W):E(f):", "CW (T):f.E(f):", "LDA (U):f.E(f):", "LDA (W):f.E(f):", "Folder::", "Inst::"]
  in  "String 6":string
  in  "E":u16(ring) items=["File::", "Date::", "Time::", "Comments::", "Chilled Water:Temp:", "Inlet_Temp:Average:", "Av:Floor:Temp", "Max:deltaT:", "X (mm)::", "Y (mm)::", "Z (mm)::", "Z (m)::", "U/Uref::", "u^2/Uref^2::", "w^2/Uref^2::", "-uw/Uref^2::", "Inlet:DeltaT:", "DeltaT::", "t^2::", "ut::", "wt::", "Grad:Ri:", "Flux:Ri:", "B-V:Freq:N", "DeltaT/DeltaTmax::", "W/Uref::", "T:thermistor:", "dT/dZ::", "dU/dZ::", "Inlet:Delta_Set:", "u'/U::", "w'/U::", "W/U::", "Location:XY:", "Location:XZ:", "U:m/s:", "W:m/s:", "u^2::", "w^2::", "Speed/Uref::", "T:cw:", "Uref::", "Flow:Meas:Time", "Profile::", "t'/T::", "t'::", "uw::", "Spires::", "Roughness::", "Z=1450:Inlet:Temp", "Z=1350:Inlet:Temp", "Z=1250:Inlet:Temp", "Z=1150:Inlet:Temp", "Z=1050:Inlet:Temp", "Z=950:Inlet:Temp", "Z=850:Inlet:Temp", "Z=750:Inlet:Temp", "Z=650:Inlet:Temp", "Z=550:Inlet:Temp", "Z=450:Inlet:Temp", "Z=350:Inlet:Temp", "Z=250:Inlet:Temp", "Z=150:Inlet:Temp", "Z=50:Inlet:Temp", "EnFlo Lab:Hygrometry:Dew Point temp", "EnFlo Lab:Hygrometry:Dew Point temp_PN", "Multi Run:Start Time:", "T cw:Offset:A", "T cw:Grad:B", "LDA (U):Standard Error:in Variance", "LDA (U):Standard Error:in Mean", "LDA (W):Standard Error:in Mean", "LDA (W):Standard Error:in Variance", "U/Uref::Err", "u^2/Uref^2::Err", "W/Uref::Err", "w^2/Uref^2::Err", "Inlet Temp::", "Inlet Setpoint::", "Inlet:Temp:Error", "Seconds:since:1st Jan", "Uni:Chilled Water:Temp", "EnFlo_Tunnel:Chilled Water:Valve Dem Pos", "EnFlo_Tunnel:Temp:Floor_Up_Y=-1585", "EnFlo_Tunnel:Temp:Floor_Up_Y=-1250", "EnFlo_Tunnel:Temp:Floor_Up_Y=-920", "EnFlo_Tunnel:Temp:Floor_Up_Y=-585", "EnFlo_Tunnel:Temp:Floor_Up_Y=-250", "EnFlo_Tunnel:Temp:Floor_Up_Y=80", "EnFlo_Tunnel:Temp:Floor_Up_Y=415", "EnFlo_Tunnel:Temp:Floor_Up_Y=750", "EnFlo_Tunnel:Temp:Floor_Up_Y=1080", "EnFlo_Tunnel:Temp:Floor_Up_Y=1415", "Raw:Data:Filename", "Z=1450:Inlet:Setpoint", "Z=1350:Inlet:Setpoint", "Z=1250:Inlet:Setpoint", "Z=1150:Inlet:Setpoint", "Z=1050:Inlet:Setpoint", "Z=950:Inlet:Setpoint", "Z=850:Inlet:Setpoint", "Z=750:Inlet:Setpoint", "Z=650:Inlet:Setpoint", "Z=550:Inlet:Setpoint", "Z=450:Inlet:Setpoint", "Z=350:Inlet:Setpoint", "Z=250:Inlet:Setpoint", "Z=150:Inlet:Setpoint", "Z=50:Inlet:Setpoint", "Freq:Hz:", "LDA (U):E(f):", "LDA (W):E(f):", "CW (T):f.E(f):", "LDA (U):f.E(f):", "LDA (W):f.E(f):", "Folder::", "Inst::"]
  in  "String 5":string
  in  "D":u16(ring) items=["File::", "Date::", "Time::", "Comments::", "Chilled Water:Temp:", "Inlet_Temp:Average:", "Av:Floor:Temp", "Max:deltaT:", "X (mm)::", "Y (mm)::", "Z (mm)::", "Z (m)::", "U/Uref::", "u^2/Uref^2::", "w^2/Uref^2::", "-uw/Uref^2::", "Inlet:DeltaT:", "DeltaT::", "t^2::", "ut::", "wt::", "Grad:Ri:", "Flux:Ri:", "B-V:Freq:N", "DeltaT/DeltaTmax::", "W/Uref::", "T:thermistor:", "dT/dZ::", "dU/dZ::", "Inlet:Delta_Set:", "u'/U::", "w'/U::", "W/U::", "Location:XY:", "Location:XZ:", "U:m/s:", "W:m/s:", "u^2::", "w^2::", "Speed/Uref::", "T:cw:", "Uref::", "Flow:Meas:Time", "Profile::", "t'/T::", "t'::", "uw::", "Spires::", "Roughness::", "Z=1450:Inlet:Temp", "Z=1350:Inlet:Temp", "Z=1250:Inlet:Temp", "Z=1150:Inlet:Temp", "Z=1050:Inlet:Temp", "Z=950:Inlet:Temp", "Z=850:Inlet:Temp", "Z=750:Inlet:Temp", "Z=650:Inlet:Temp", "Z=550:Inlet:Temp", "Z=450:Inlet:Temp", "Z=350:Inlet:Temp", "Z=250:Inlet:Temp", "Z=150:Inlet:Temp", "Z=50:Inlet:Temp", "EnFlo Lab:Hygrometry:Dew Point temp", "EnFlo Lab:Hygrometry:Dew Point temp_PN", "Multi Run:Start Time:", "T cw:Offset:A", "T cw:Grad:B", "LDA (U):Standard Error:in Variance", "LDA (U):Standard Error:in Mean", "LDA (W):Standard Error:in Mean", "LDA (W):Standard Error:in Variance", "U/Uref::Err", "u^2/Uref^2::Err", "W/Uref::Err", "w^2/Uref^2::Err", "Inlet Temp::", "Inlet Setpoint::", "Inlet:Temp:Error", "Seconds:since:1st Jan", "Uni:Chilled Water:Temp", "EnFlo_Tunnel:Chilled Water:Valve Dem Pos", "EnFlo_Tunnel:Temp:Floor_Up_Y=-1585", "EnFlo_Tunnel:Temp:Floor_Up_Y=-1250", "EnFlo_Tunnel:Temp:Floor_Up_Y=-920", "EnFlo_Tunnel:Temp:Floor_Up_Y=-585", "EnFlo_Tunnel:Temp:Floor_Up_Y=-250", "EnFlo_Tunnel:Temp:Floor_Up_Y=80", "EnFlo_Tunnel:Temp:Floor_Up_Y=415", "EnFlo_Tunnel:Temp:Floor_Up_Y=750", "EnFlo_Tunnel:Temp:Floor_Up_Y=1080", "EnFlo_Tunnel:Temp:Floor_Up_Y=1415", "Raw:Data:Filename", "Z=1450:Inlet:Setpoint", "Z=1350:Inlet:Setpoint", "Z=1250:Inlet:Setpoint", "Z=1150:Inlet:Setpoint", "Z=1050:Inlet:Setpoint", "Z=950:Inlet:Setpoint", "Z=850:Inlet:Setpoint", "Z=750:Inlet:Setpoint", "Z=650:Inlet:Setpoint", "Z=550:Inlet:Setpoint", "Z=450:Inlet:Setpoint", "Z=350:Inlet:Setpoint", "Z=250:Inlet:Setpoint", "Z=150:Inlet:Setpoint", "Z=50:Inlet:Setpoint", "Freq:Hz:", "LDA (U):E(f):", "LDA (W):E(f):", "CW (T):f.E(f):", "LDA (U):f.E(f):", "LDA (W):f.E(f):", "Folder::", "Inst::"]
  in  "String 4":string
  in  "C":u16(ring) items=["File::", "Date::", "Time::", "Comments::", "Chilled Water:Temp:", "Inlet_Temp:Average:", "Av:Floor:Temp", "Max:deltaT:", "X (mm)::", "Y (mm)::", "Z (mm)::", "Z (m)::", "U/Uref::", "u^2/Uref^2::", "w^2/Uref^2::", "-uw/Uref^2::", "Inlet:DeltaT:", "DeltaT::", "t^2::", "ut::", "wt::", "Grad:Ri:", "Flux:Ri:", "B-V:Freq:N", "DeltaT/DeltaTmax::", "W/Uref::", "T:thermistor:", "dT/dZ::", "dU/dZ::", "Inlet:Delta_Set:", "u'/U::", "w'/U::", "W/U::", "Location:XY:", "Location:XZ:", "U:m/s:", "W:m/s:", "u^2::", "w^2::", "Speed/Uref::", "T:cw:", "Uref::", "Flow:Meas:Time", "Profile::", "t'/T::", "t'::", "uw::", "Spires::", "Roughness::", "Z=1450:Inlet:Temp", "Z=1350:Inlet:Temp", "Z=1250:Inlet:Temp", "Z=1150:Inlet:Temp", "Z=1050:Inlet:Temp", "Z=950:Inlet:Temp", "Z=850:Inlet:Temp", "Z=750:Inlet:Temp", "Z=650:Inlet:Temp", "Z=550:Inlet:Temp", "Z=450:Inlet:Temp", "Z=350:Inlet:Temp", "Z=250:Inlet:Temp", "Z=150:Inlet:Temp", "Z=50:Inlet:Temp", "EnFlo Lab:Hygrometry:Dew Point temp", "EnFlo Lab:Hygrometry:Dew Point temp_PN", "Multi Run:Start Time:", "T cw:Offset:A", "T cw:Grad:B", "LDA (U):Standard Error:in Variance", "LDA (U):Standard Error:in Mean", "LDA (W):Standard Error:in Mean", "LDA (W):Standard Error:in Variance", "U/Uref::Err", "u^2/Uref^2::Err", "W/Uref::Err", "w^2/Uref^2::Err", "Inlet Temp::", "Inlet Setpoint::", "Inlet:Temp:Error", "Seconds:since:1st Jan", "Uni:Chilled Water:Temp", "EnFlo_Tunnel:Chilled Water:Valve Dem Pos", "EnFlo_Tunnel:Temp:Floor_Up_Y=-1585", "EnFlo_Tunnel:Temp:Floor_Up_Y=-1250", "EnFlo_Tunnel:Temp:Floor_Up_Y=-920", "EnFlo_Tunnel:Temp:Floor_Up_Y=-585", "EnFlo_Tunnel:Temp:Floor_Up_Y=-250", "EnFlo_Tunnel:Temp:Floor_Up_Y=80", "EnFlo_Tunnel:Temp:Floor_Up_Y=415", "EnFlo_Tunnel:Temp:Floor_Up_Y=750", "EnFlo_Tunnel:Temp:Floor_Up_Y=1080", "EnFlo_Tunnel:Temp:Floor_Up_Y=1415", "Raw:Data:Filename", "Z=1450:Inlet:Setpoint", "Z=1350:Inlet:Setpoint", "Z=1250:Inlet:Setpoint", "Z=1150:Inlet:Setpoint", "Z=1050:Inlet:Setpoint", "Z=950:Inlet:Setpoint", "Z=850:Inlet:Setpoint", "Z=750:Inlet:Setpoint", "Z=650:Inlet:Setpoint", "Z=550:Inlet:Setpoint", "Z=450:Inlet:Setpoint", "Z=350:Inlet:Setpoint", "Z=250:Inlet:Setpoint", "Z=150:Inlet:Setpoint", "Z=50:Inlet:Setpoint", "Freq:Hz:", "LDA (U):E(f):", "LDA (W):E(f):", "CW (T):f.E(f):", "LDA (U):f.E(f):", "LDA (W):f.E(f):", "Folder::", "Inst::"]
  in  "String 3":string
  in  "B":u16(ring) items=["File::", "Date::", "Time::", "Comments::", "Chilled Water:Temp:", "Inlet_Temp:Average:", "Av:Floor:Temp", "Max:deltaT:", "X (mm)::", "Y (mm)::", "Z (mm)::", "Z (m)::", "U/Uref::", "u^2/Uref^2::", "w^2/Uref^2::", "-uw/Uref^2::", "Inlet:DeltaT:", "DeltaT::", "t^2::", "ut::", "wt::", "Grad:Ri:", "Flux:Ri:", "B-V:Freq:N", "DeltaT/DeltaTmax::", "W/Uref::", "T:thermistor:", "dT/dZ::", "dU/dZ::", "Inlet:Delta_Set:", "u'/U::", "w'/U::", "W/U::", "Location:XY:", "Location:XZ:", "U:m/s:", "W:m/s:", "u^2::", "w^2::", "Speed/Uref::", "T:cw:", "Uref::", "Flow:Meas:Time", "Profile::", "t'/T::", "t'::", "uw::", "Spires::", "Roughness::", "Z=1450:Inlet:Temp", "Z=1350:Inlet:Temp", "Z=1250:Inlet:Temp", "Z=1150:Inlet:Temp", "Z=1050:Inlet:Temp", "Z=950:Inlet:Temp", "Z=850:Inlet:Temp", "Z=750:Inlet:Temp", "Z=650:Inlet:Temp", "Z=550:Inlet:Temp", "Z=450:Inlet:Temp", "Z=350:Inlet:Temp", "Z=250:Inlet:Temp", "Z=150:Inlet:Temp", "Z=50:Inlet:Temp", "EnFlo Lab:Hygrometry:Dew Point temp", "EnFlo Lab:Hygrometry:Dew Point temp_PN", "Multi Run:Start Time:", "T cw:Offset:A", "T cw:Grad:B", "LDA (U):Standard Error:in Variance", "LDA (U):Standard Error:in Mean", "LDA (W):Standard Error:in Mean", "LDA (W):Standard Error:in Variance", "U/Uref::Err", "u^2/Uref^2::Err", "W/Uref::Err", "w^2/Uref^2::Err", "Inlet Temp::", "Inlet Setpoint::", "Inlet:Temp:Error", "Seconds:since:1st Jan", "Uni:Chilled Water:Temp", "EnFlo_Tunnel:Chilled Water:Valve Dem Pos", "EnFlo_Tunnel:Temp:Floor_Up_Y=-1585", "EnFlo_Tunnel:Temp:Floor_Up_Y=-1250", "EnFlo_Tunnel:Temp:Floor_Up_Y=-920", "EnFlo_Tunnel:Temp:Floor_Up_Y=-585", "EnFlo_Tunnel:Temp:Floor_Up_Y=-250", "EnFlo_Tunnel:Temp:Floor_Up_Y=80", "EnFlo_Tunnel:Temp:Floor_Up_Y=415", "EnFlo_Tunnel:Temp:Floor_Up_Y=750", "EnFlo_Tunnel:Temp:Floor_Up_Y=1080", "EnFlo_Tunnel:Temp:Floor_Up_Y=1415", "Raw:Data:Filename", "Z=1450:Inlet:Setpoint", "Z=1350:Inlet:Setpoint", "Z=1250:Inlet:Setpoint", "Z=1150:Inlet:Setpoint", "Z=1050:Inlet:Setpoint", "Z=950:Inlet:Setpoint", "Z=850:Inlet:Setpoint", "Z=750:Inlet:Setpoint", "Z=650:Inlet:Setpoint", "Z=550:Inlet:Setpoint", "Z=450:Inlet:Setpoint", "Z=350:Inlet:Setpoint", "Z=250:Inlet:Setpoint", "Z=150:Inlet:Setpoint", "Z=50:Inlet:Setpoint", "Freq:Hz:", "LDA (U):E(f):", "LDA (W):E(f):", "CW (T):f.E(f):", "LDA (U):f.E(f):", "LDA (W):f.E(f):", "Folder::", "Inst::"]
  in  "String 2":string
  in  "A":u16(ring) items=["File::", "Date::", "Time::", "Comments::", "Chilled Water:Temp:", "Inlet_Temp:Average:", "Av:Floor:Temp", "Max:deltaT:", "X (mm)::", "Y (mm)::", "Z (mm)::", "Z (m)::", "U/Uref::", "u^2/Uref^2::", "w^2/Uref^2::", "-uw/Uref^2::", "Inlet:DeltaT:", "DeltaT::", "t^2::", "ut::", "wt::", "Grad:Ri:", "Flux:Ri:", "B-V:Freq:N", "DeltaT/DeltaTmax::", "W/Uref::", "T:thermistor:", "dT/dZ::", "dU/dZ::", "Inlet:Delta_Set:", "u'/U::", "w'/U::", "W/U::", "Location:XY:", "Location:XZ:", "U:m/s:", "W:m/s:", "u^2::", "w^2::", "Speed/Uref::", "T:cw:", "Uref::", "Flow:Meas:Time", "Profile::", "t'/T::", "t'::", "uw::", "Spires::", "Roughness::", "Z=1450:Inlet:Temp", "Z=1350:Inlet:Temp", "Z=1250:Inlet:Temp", "Z=1150:Inlet:Temp", "Z=1050:Inlet:Temp", "Z=950:Inlet:Temp", "Z=850:Inlet:Temp", "Z=750:Inlet:Temp", "Z=650:Inlet:Temp", "Z=550:Inlet:Temp", "Z=450:Inlet:Temp", "Z=350:Inlet:Temp", "Z=250:Inlet:Temp", "Z=150:Inlet:Temp", "Z=50:Inlet:Temp", "EnFlo Lab:Hygrometry:Dew Point temp", "EnFlo Lab:Hygrometry:Dew Point temp_PN", "Multi Run:Start Time:", "T cw:Offset:A", "T cw:Grad:B", "LDA (U):Standard Error:in Variance", "LDA (U):Standard Error:in Mean", "LDA (W):Standard Error:in Mean", "LDA (W):Standard Error:in Variance", "U/Uref::Err", "u^2/Uref^2::Err", "W/Uref::Err", "w^2/Uref^2::Err", "Inlet Temp::", "Inlet Setpoint::", "Inlet:Temp:Error", "Seconds:since:1st Jan", "Uni:Chilled Water:Temp", "EnFlo_Tunnel:Chilled Water:Valve Dem Pos", "EnFlo_Tunnel:Temp:Floor_Up_Y=-1585", "EnFlo_Tunnel:Temp:Floor_Up_Y=-1250", "EnFlo_Tunnel:Temp:Floor_Up_Y=-920", "EnFlo_Tunnel:Temp:Floor_Up_Y=-585", "EnFlo_Tunnel:Temp:Floor_Up_Y=-250", "EnFlo_Tunnel:Temp:Floor_Up_Y=80", "EnFlo_Tunnel:Temp:Floor_Up_Y=415", "EnFlo_Tunnel:Temp:Floor_Up_Y=750", "EnFlo_Tunnel:Temp:Floor_Up_Y=1080", "EnFlo_Tunnel:Temp:Floor_Up_Y=1415", "Raw:Data:Filename", "Z=1450:Inlet:Setpoint", "Z=1350:Inlet:Setpoint", "Z=1250:Inlet:Setpoint", "Z=1150:Inlet:Setpoint", "Z=1050:Inlet:Setpoint", "Z=950:Inlet:Setpoint", "Z=850:Inlet:Setpoint", "Z=750:Inlet:Setpoint", "Z=650:Inlet:Setpoint", "Z=550:Inlet:Setpoint", "Z=450:Inlet:Setpoint", "Z=350:Inlet:Setpoint", "Z=250:Inlet:Setpoint", "Z=150:Inlet:Setpoint", "Z=50:Inlet:Setpoint", "Freq:Hz:", "LDA (U):E(f):", "LDA (W):E(f):", "CW (T):f.E(f):", "LDA (U):f.E(f):", "LDA (W):f.E(f):", "Folder::", "Inst::"]
  in  "String 1":string
  in  "Reset":bool
  in  "Number of Variables":i32
  in  "OK":bool
  # "> 20  or  <20  or  =hello   or \n£hello  (not equal to hello)"
  # "<<Characters_to_Match>>  <<Replace_Whole_String_with_this>>"
  # "<<Channel_Name>> contains <<Characters to match>> or\n<<Channel_Name>> does not contain <<Characters to match>>"
  # "<<Channel_Name_A>> + <<Channel_Name_B>> or\nConcatenate <<Channel_Name_A>> and <<Channel_Name_B>>"
  # "> 20  or  <20  or  =hello   or \n£hello  (not equal to hello)"
  # "<<Characters_to_Match>>  <<Replace_Whole_String_with_this>>"
  # "<<Channel_Name>> contains <<Characters to match>> or\n<<Channel_Name>> does not contain <<Characters to match>>"
  # "<<Channel_Name_A>> + <<Channel_Name_B>> or\nConcatenate <<Channel_Name_A>> and <<Channel_Name_B>>"
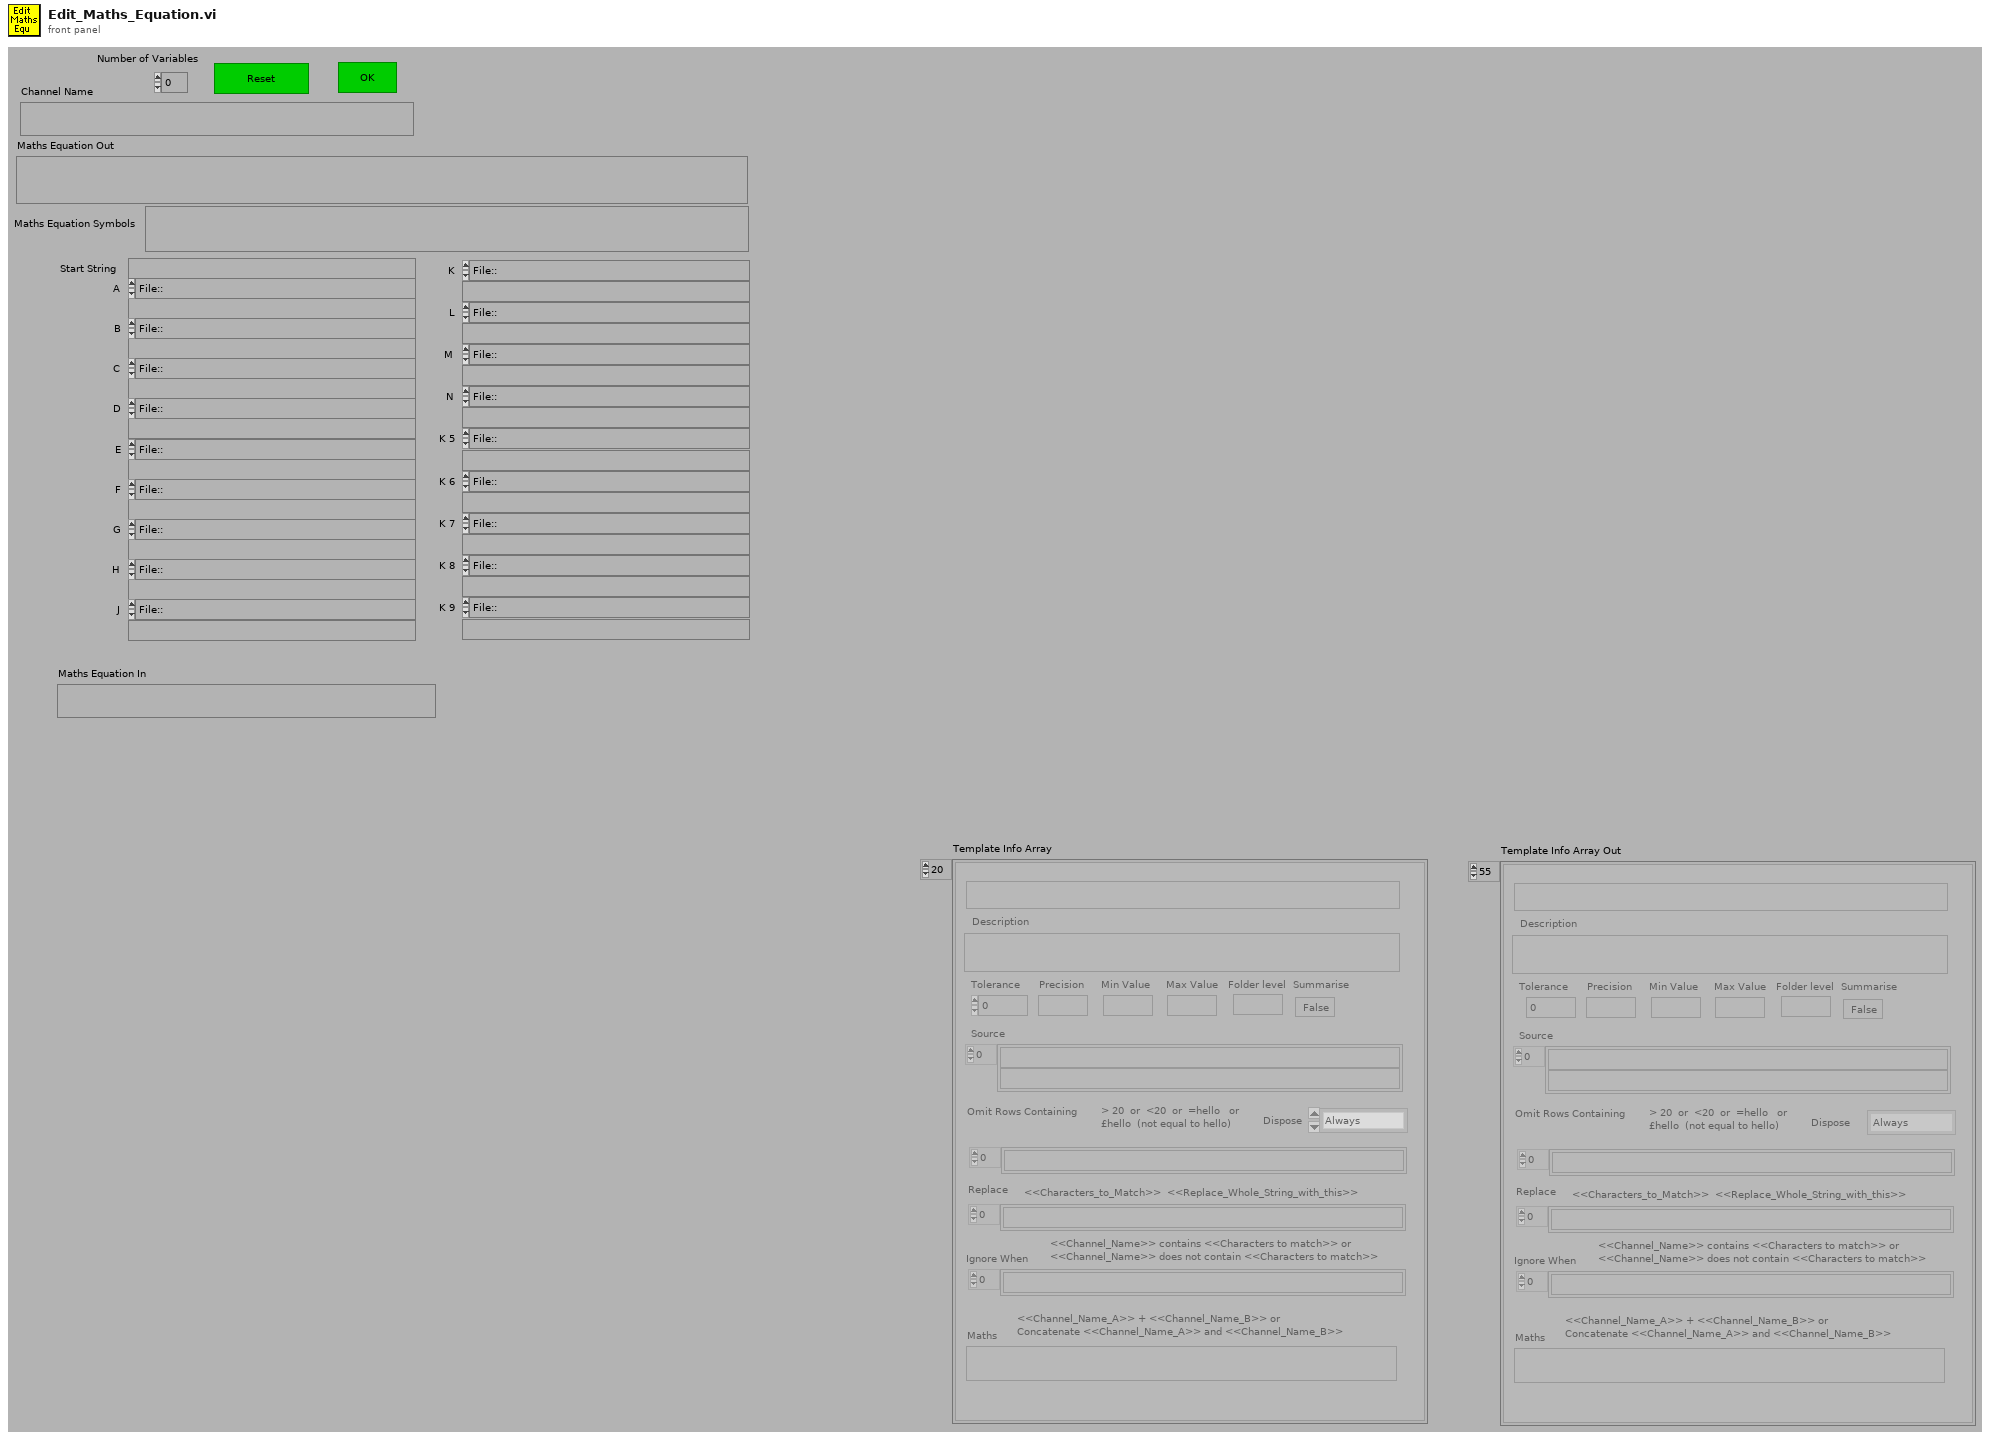
[diagram p1: front panel]
types:
  T1 = typedef "File_Template_Clus.ctl" = cluster{"Template Channel Name":string, "Description":string, "Tolerance":dbl, "Precision":string, "Folder level":string, "Source":string[], "Replace":string[], "Summarise":bool, "Min Value":string, "Maths":string, "Omit Rows Containing":string[], "Ignore When":string[], "Max Value":string, "Dispose":T2}
  T2 = typedef "Dispose_Channel.ctl" = enum16{"Always", "If Blank", "Never"}
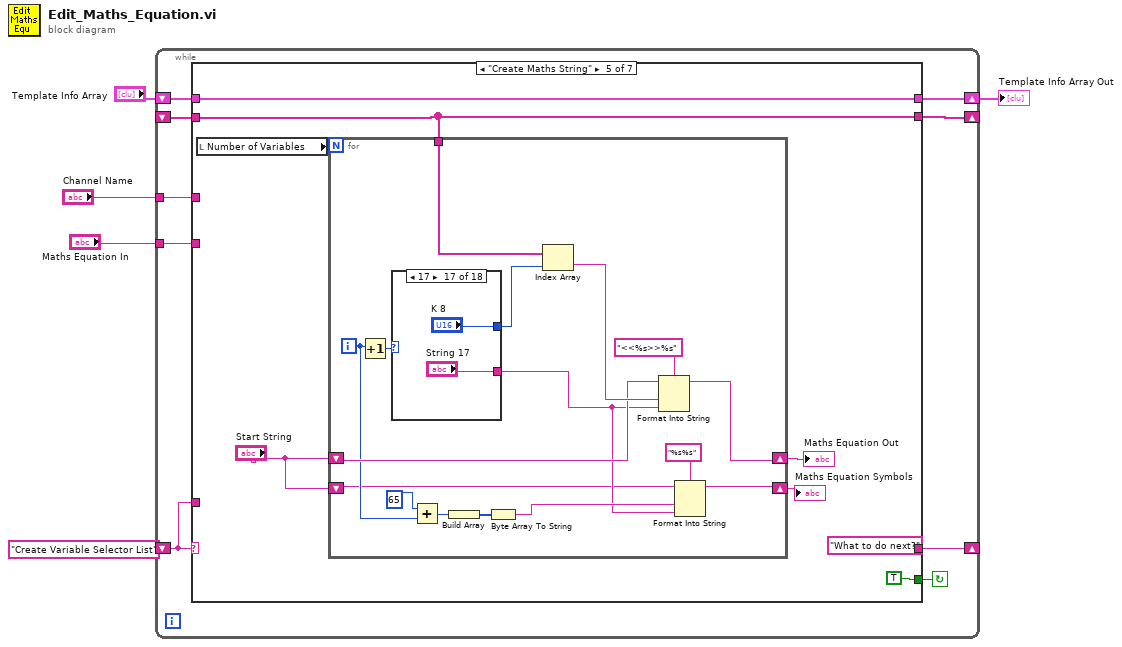
[diagram p0: block diagram]
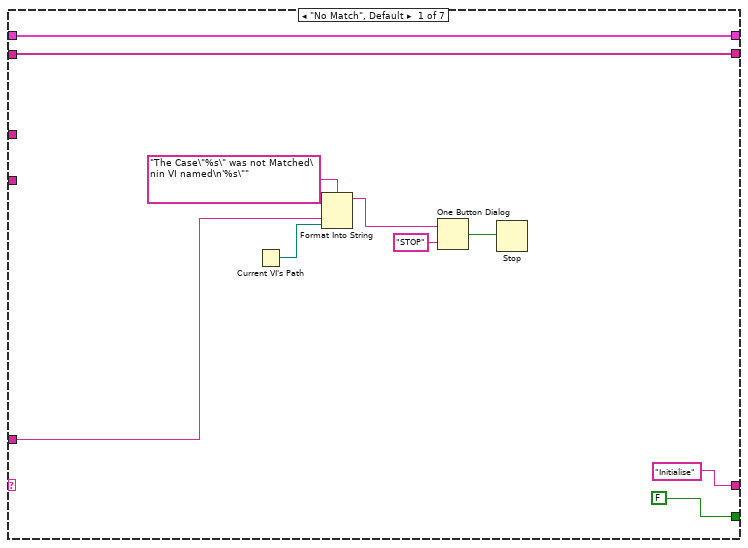
[diagram p2: hidden frame]
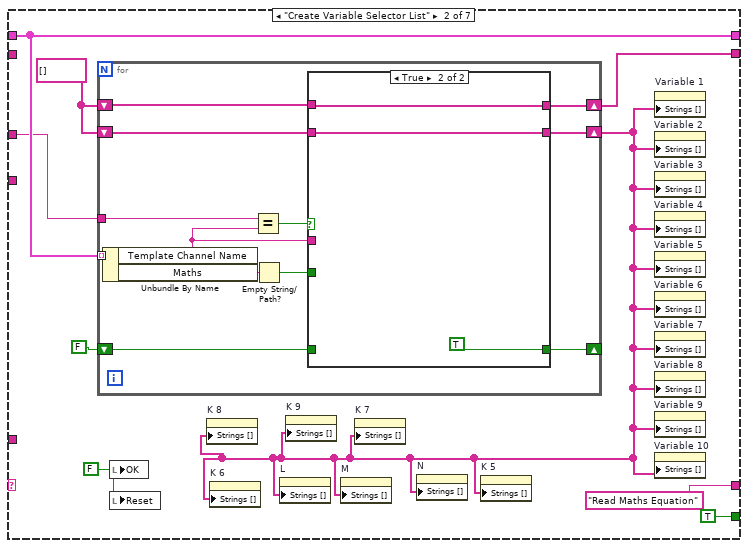
[diagram p3: hidden frame]
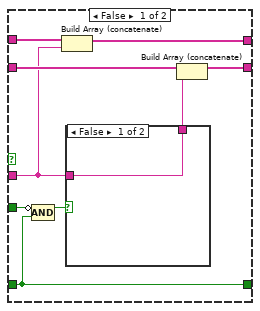
[diagram p4: hidden frame]
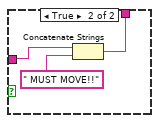
[diagram p5: hidden frame]
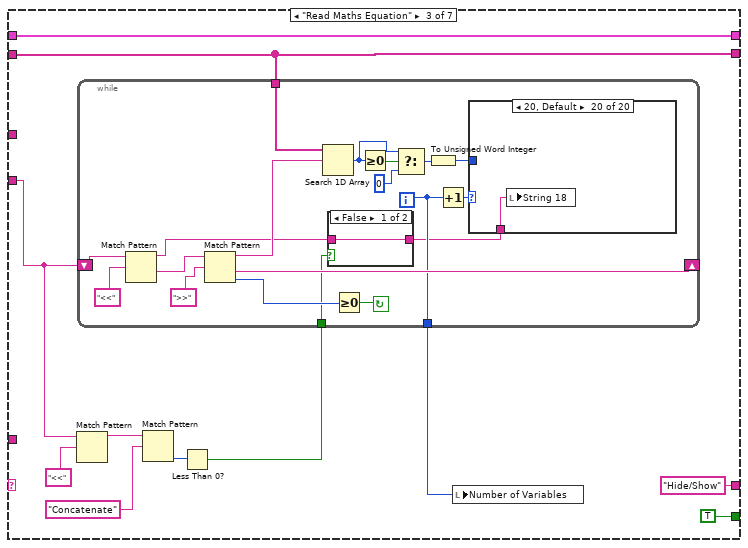
[diagram p6: hidden frame]
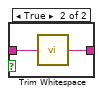
[diagram p7: hidden frame]
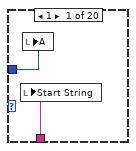
[diagram p8: hidden frame]
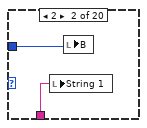
[diagram p9: hidden frame]
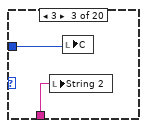
[diagram p10: hidden frame]
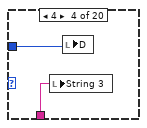
[diagram p11: hidden frame]
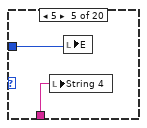
[diagram p12: hidden frame]
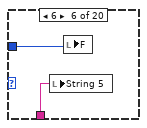
[diagram p13: hidden frame]
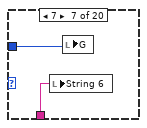
[diagram p14: hidden frame]
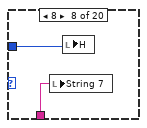
[diagram p15: hidden frame]
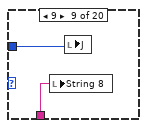
[diagram p16: hidden frame]
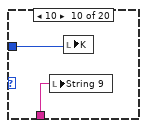
[diagram p17: hidden frame]
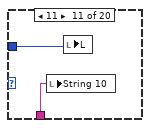
[diagram p18: hidden frame]
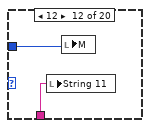
[diagram p19: hidden frame]
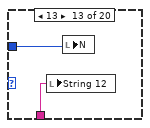
[diagram p20: hidden frame]
diagram:
  n1 = while {
    tunnel: "Channel Name" -> [w6]
    tunnel: "Maths Equation In" -> [w7]
    shift-left: _ -> [w8]
    shift-right: [w9] -> _
    shift-left: "Template Info Array" -> [w10]
    shift-right: [w11] -> w3
    shift-left: "Create Variable Selector List" -> [w12]
    shift-right: [w13] -> _
    stop <- w14 continue-if-true
    n2 = case shown="\"Create Maths String\"" w12 {
      tunnel: [FALSE TRUE TRUE TRUE TRUE TRUE FALSE] -> w14
      tunnel: ["Initialise" "Read Maths Equation" "Hide/Show" "Create Maths String" "What to do next?" w221 "End"] -> w13
      tunnel: w12 -> [w19 _ _ _ _ _ _]
      tunnel: [w16 w32 w71 w136 w165 w231 w240] -> w11
      tunnel: w10 -> [w16 w32 w71 w136 w165 w231 w240]
      tunnel: [w15 w30 w70 w135 w163 w225 w239] -> w9
      tunnel: w8 -> [w15 _ w70 w135 w163 w225 w239]
      tunnel: w7 -> [_ _ w66 _ _ _ _]
      tunnel: w6 -> [_ w31 _ _ _ _ _]
      frame "No Match", Default {
        n3 = Current VI's Path() -> (path=w18:path)
        n4 = Format Into String(format string="The Case\"%s\" was not Matched\nin VI named\n'%s\"" ("Format String"), w19, w18) -> (resulting string=w22:string)  [unwired: 2 in, 1 out]
        n5 = One Button Dialog(message=w22, button name ("OK")="STOP") -> (true=w20:bool)
        n6 = Stop(stop? (T)=w20) -> ()
      }
      frame "Create Variable Selector List" {
        w26 = FALSE ("OK")
        w28 = string[] []
        n7 = for {
          shift-right: [w40] -> w30
          shift-left: w28 -> [w42]
          shift-right: [w36] -> w25
          shift-left: w28 -> [w37]
          tunnel: w32 -> [w45] mode=indexing
          tunnel: w31 -> [w44]
          shift-right: [w35] -> _
          shift-left: FALSE -> [w34]
          n8 = Unbundle By Name(w45) -> ("Template Channel Name"=w41:string, "Maths"=w39:string)
          n9 = Equal?(x=w44, y=w41) -> (x = y?=w43:bool)
          n10 = Empty String/Path?(string/path=w39) -> (empty?=w38:bool)
          n11 = case shown="True" w43 {
            tunnel: w42 -> [w54 w60]
            tunnel: w41 -> [w49 _]
            tunnel: [w53 w60] -> w40
            tunnel: w38 -> [w48 _]
            tunnel: w37 -> [w52 w59]
            tunnel: [w51 w59] -> w36
            tunnel: [w46 TRUE] -> w35
            tunnel: w34 -> [w46 _]
            frame False {
              n12 = Compound Arithmetic op=AND(invert w48, w46) -> (w47:bool)
              n13 = Build Array (concatenate)(w54, w49) -> (w53:string[])
              n14 = case shown="False" w47 {
                tunnel: [w55 w57] -> w50
                tunnel: w49 -> [w55 w58]
                frame False {
                }
                frame True {
                  n15 = Concatenate Strings(w58, " MUST MOVE!!" ("Substring")) -> (w57:string)
                }
              }
              n16 = Build Array (concatenate)(w52, w50) -> (w51:string[])
            }
            frame True {
            }
          }
        }
        n17 = local write "OK"(w26) -> ()
        n18 = local write "Reset"(w26) -> ()
        n19 = property on="K 8" class="Ring (strict)"("Strings []"=w25) -> ()  [unwired: 2 in, 2 out]
        n20 = property on="K 6" class="Ring (strict)"("Strings []"=w25) -> ()  [unwired: 2 in, 2 out]
        n21 = property on="L" class="Ring (strict)"("Strings []"=w25) -> ()  [unwired: 2 in, 2 out]
        n22 = property on="K 9" class="Ring (strict)"("Strings []"=w25) -> ()  [unwired: 2 in, 2 out]
        n23 = property on="M" class="Ring (strict)"("Strings []"=w25) -> ()  [unwired: 2 in, 2 out]
        n24 = property on="K 7" class="Ring (strict)"("Strings []"=w25) -> ()  [unwired: 2 in, 2 out]
        n25 = property on="N" class="Ring (strict)"("Strings []"=w25) -> ()  [unwired: 2 in, 2 out]
        n26 = property on="K 5" class="Ring (strict)"("Strings []"=w25) -> ()  [unwired: 2 in, 2 out]
        n27 = property on="Variable 1" class="Ring (strict)"("Strings []"=w25) -> ()  [unwired: 2 in, 2 out]
        n28 = property on="Variable 2" class="Ring (strict)"("Strings []"=w25) -> ()  [unwired: 2 in, 2 out]
        n29 = property on="Variable 3" class="Ring (strict)"("Strings []"=w25) -> ()  [unwired: 2 in, 2 out]
        n30 = property on="Variable 4" class="Ring (strict)"("Strings []"=w25) -> ()  [unwired: 2 in, 2 out]
        n31 = property on="Variable 5" class="Ring (strict)"("Strings []"=w25) -> ()  [unwired: 2 in, 2 out]
        n32 = property on="Variable 6" class="Ring (strict)"("Strings []"=w25) -> ()  [unwired: 2 in, 2 out]
        n33 = property on="Variable 7" class="Ring (strict)"("Strings []"=w25) -> ()  [unwired: 2 in, 2 out]
        n34 = property on="Variable 8" class="Ring (strict)"("Strings []"=w25) -> ()  [unwired: 2 in, 2 out]
        n35 = property on="Variable 9" class="Ring (strict)"("Strings []"=w25) -> ()  [unwired: 2 in, 2 out]
        n36 = property on="Variable 10" class="Ring (strict)"("Strings []"=w25) -> ()  [unwired: 2 in, 2 out]
      }
      frame "Read Maths Equation" {
        n37 = Match Pattern(string=w66, regular expression="<<") -> (before substring=w65:string)  [unwired: 4 out]
        n38 = Match Pattern(string=w65, regular expression="Concatenate") -> (offset past match=w63:i32)  [unwired: 4 out]
        n39 = Less Than 0?(x=w63) -> (x < 0?=w62:bool)
        n40 = while {
          tunnel: [w79] -> w69
          tunnel: w70 -> [w88]
          shift-left: w66 -> [w91]
          shift-right: [w81] -> _
          tunnel: w62 -> [w73]
          i -> [w79]
          stop <- w89 continue-if-true
          n41 = Match Pattern(string=w91, regular expression="<<") -> (before substring=w77:string, after substring=w90:string)  [unwired: 3 out]
          n42 = Match Pattern(string=w90, regular expression=">>") -> (before substring=w87:string, after substring=w81:string, offset past match=w80:i32)  [unwired: 2 out]
          n43 = Search 1D Array(1D array=w88, element=w87) -> (index of element=w85:i32)  [unwired: 1 out]
          n44 = case shown="False" w73 {
            tunnel: w77 -> [w92 w94]
            tunnel: [w92 w93] -> w76
            frame False {
            }
            frame True {
              n45 = call <vilib>:"Trim Whitespace.vi"("string"=w94) -> ("trimmed string"=w93:string)  [unwired: 1 in]
            }
          }
          n46 = Greater Or Equal To 0?(x=w80) -> (x >= 0?=w89:bool)
          n47 = Greater Or Equal To 0?(x=w85) -> (x >= 0?=w86:bool)
          n48 = Select(t=w85, s=w86, f=0) -> (s? t:f=w82:i32)
          n49 = To Unsigned Word Integer(number=w82) -> (unsigned 16bit integer=w78:u16)
          n50 = Increment(x=w79) -> (x+1=w83:i32)
          n51 = case shown="20, Default" w83 {
            tunnel: w78 -> [w96 w98 w100 w102 w104 w106 w108 w110 w112 w114 w116 w118 w120 w122 w124 w125 _ w127 w129 _]
            tunnel: w76 -> [w95 w97 w99 w101 w103 w105 w107 w109 w111 w113 w115 w117 w119 w121 w123 w126 _ w128 w130 w131]
            frame 1 {
              n52 = local write "Start String"(w95) -> ()
              n53 = local write "A"(w96) -> ()
            }
            frame 2 {
              n54 = local write "String 1"(w97) -> ()
              n55 = local write "B"(w98) -> ()
            }
            frame 3 {
              n56 = local write "String 2"(w99) -> ()
              n57 = local write "C"(w100) -> ()
            }
            frame 4 {
              n58 = local write "String 3"(w101) -> ()
              n59 = local write "D"(w102) -> ()
            }
            frame 5 {
              n60 = local write "String 4"(w103) -> ()
              n61 = local write "E"(w104) -> ()
            }
            frame 6 {
              n62 = local write "String 5"(w105) -> ()
              n63 = local write "F"(w106) -> ()
            }
            frame 7 {
              n64 = local write "String 6"(w107) -> ()
              n65 = local write "G"(w108) -> ()
            }
            frame 8 {
              n66 = local write "String 7"(w109) -> ()
              n67 = local write "H"(w110) -> ()
            }
            frame 9 {
              n68 = local write "String 8"(w111) -> ()
              n69 = local write "J"(w112) -> ()
            }
            frame 10 {
              n70 = local write "String 9"(w113) -> ()
              n71 = local write "K"(w114) -> ()
            }
            frame 11 {
              n72 = local write "String 10"(w115) -> ()
              n73 = local write "L"(w116) -> ()
            }
            frame 12 {
              n74 = local write "String 11"(w117) -> ()
              n75 = local write "M"(w118) -> ()
            }
            frame 13 {
              n76 = local write "String 12"(w119) -> ()
              n77 = local write "N"(w120) -> ()
            }
            frame 14 {
              n78 = local write "String 13"(w121) -> ()
              n79 = local write "K 5"(w122) -> ()
            }
            frame 15 {
              n80 = local write "String 14"(w123) -> ()
              n81 = local write "K 6"(w124) -> ()
            }
            frame 16 {
              n82 = local write "String 15"(w126) -> ()
              n83 = local write "K 7"(w125) -> ()
            }
            frame 17 {
            }
            frame 18 {
              n84 = local write "String 16"(w128) -> ()
              n85 = local write "K 8"(w127) -> ()
            }
            frame 19 {
              n86 = local write "String 17"(w130) -> ()
              n87 = local write "K 9"(w129) -> ()
            }
            frame 20, Default {
              n88 = local write "String 18"(w131) -> ()
            }
          }
        }
        n89 = local write "Number of Variables"(w69) -> ()
      }
      frame "Hide/Show" {
        n90 = for {
          N: 19 -> [_]
          tunnel: "Number of Variables" -> [w139]
          i -> [w141]
          n91 = Increment(x=w141) -> (x+1=w140:i32)
          n92 = Less Or Equal?(x=w140, y=w139) -> (x <= y?=w138:bool)
          n93 = case shown="0, Default" w140 {
            tunnel: w138 -> [_ w142 w143 w144 w145 w146 w147 w148 w149 w150 w151 w152 w153 w154 w155 w156 w157 w158 w159]
            frame 0, Default {
            }
            frame 1 {
              n94 = property on="Variable 1" class="Ring (strict)"("Visible"=w142) -> ()  [unwired: 2 in, 2 out]
              n95 = property on="String 1" class="Str"("Visible"=w142) -> ()  [unwired: 2 in, 2 out]
            }
            frame 2 {
              n96 = property on="Variable 2" class="Ring (strict)"("Visible"=w143) -> ()  [unwired: 2 in, 2 out]
              n97 = property on="String 2" class="Str"("Visible"=w143) -> ()  [unwired: 2 in, 2 out]
            }
            frame 3 {
              n98 = property on="Variable 3" class="Ring (strict)"("Visible"=w144) -> ()  [unwired: 2 in, 2 out]
              n99 = property on="String 3" class="Str"("Visible"=w144) -> ()  [unwired: 2 in, 2 out]
            }
            frame 4 {
              n100 = property on="String 4" class="Str"("Visible"=w145) -> ()  [unwired: 2 in, 2 out]
              n101 = property on="Variable 4" class="Ring (strict)"("Visible"=w145) -> ()  [unwired: 2 in, 2 out]
            }
            frame 5 {
              n102 = property on="String 5" class="Str"("Visible"=w146) -> ()  [unwired: 2 in, 2 out]
              n103 = property on="Variable 5" class="Ring (strict)"("Visible"=w146) -> ()  [unwired: 2 in, 2 out]
            }
            frame 6 {
              n104 = property on="String 6" class="Str"("Visible"=w147) -> ()  [unwired: 2 in, 2 out]
              n105 = property on="Variable 6" class="Ring (strict)"("Visible"=w147) -> ()  [unwired: 2 in, 2 out]
            }
            frame 7 {
              n106 = property on="Variable 7" class="Ring (strict)"("Visible"=w148) -> ()  [unwired: 2 in, 2 out]
              n107 = property on="String 7" class="Str"("Visible"=w148) -> ()  [unwired: 2 in, 2 out]
            }
            frame 8 {
              n108 = property on="String 8" class="Str"("Visible"=w149) -> ()  [unwired: 2 in, 2 out]
              n109 = property on="Variable 8" class="Ring (strict)"("Visible"=w149) -> ()  [unwired: 2 in, 2 out]
            }
            frame 9 {
              n110 = property on="String 9" class="Str"("Visible"=w150) -> ()  [unwired: 2 in, 2 out]
              n111 = property on="Variable 9" class="Ring (strict)"("Visible"=w150) -> ()  [unwired: 2 in, 2 out]
            }
            frame 10 {
              n112 = property on="Variable 10" class="Ring (strict)"("Visible"=w151) -> ()  [unwired: 2 in, 2 out]
              n113 = property on="String 10" class="Str"("Visible"=w151) -> ()  [unwired: 2 in, 2 out]
            }
            frame 11 {
              n114 = property on="L" class="Ring (strict)"("Visible"=w152) -> ()  [unwired: 2 in, 2 out]
              n115 = property on="String 11" class="Str"("Visible"=w152) -> ()  [unwired: 2 in, 2 out]
            }
            frame 12 {
              n116 = property on="M" class="Ring (strict)"("Visible"=w153) -> ()  [unwired: 2 in, 2 out]
              n117 = property on="String 12" class="Str"("Visible"=w153) -> ()  [unwired: 2 in, 2 out]
            }
            frame 13 {
              n118 = property on="N" class="Ring (strict)"("Visible"=w154) -> ()  [unwired: 2 in, 2 out]
              n119 = property on="String 13" class="Str"("Visible"=w154) -> ()  [unwired: 2 in, 2 out]
            }
            frame 14 {
              n120 = property on="K 5" class="Ring (strict)"("Visible"=w155) -> ()  [unwired: 2 in, 2 out]
              n121 = property on="String 14" class="Str"("Visible"=w155) -> ()  [unwired: 2 in, 2 out]
            }
            frame 15 {
              n122 = property on="K 6" class="Ring (strict)"("Visible"=w156) -> ()  [unwired: 2 in, 2 out]
              n123 = property on="String 15" class="Str"("Visible"=w156) -> ()  [unwired: 2 in, 2 out]
            }
            frame 16 {
              n124 = property on="K 7" class="Ring (strict)"("Visible"=w157) -> ()  [unwired: 2 in, 2 out]
              n125 = property on="String 16" class="Str"("Visible"=w157) -> ()  [unwired: 2 in, 2 out]
            }
            frame 17 {
              n126 = property on="K 8" class="Ring (strict)"("Visible"=w158) -> ()  [unwired: 2 in, 2 out]
              n127 = property on="String 17" class="Str"("Visible"=w158) -> ()  [unwired: 2 in, 2 out]
            }
            frame 18 {
              n128 = property on="K 9" class="Ring (strict)"("Visible"=w159) -> ()  [unwired: 2 in, 2 out]
              n129 = property on="String 18" class="Str"("Visible"=w159) -> ()  [unwired: 2 in, 2 out]
            }
          }
        }
      }
      frame "Create Maths String" {
        n130 = local read "Number of Variables"() -> (w164:i32)
        n131 = for {
          N: w164 -> [_]
          shift-right: [w178] -> w162
          shift-left: "Start String" -> [w179]
          tunnel: w163 -> [w183]
          shift-right: [w168] -> w160
          shift-left: "Start String" -> [w169]
          i -> [w173]
          n132 = Increment(x=w173) -> (x+1=w181:i32)
          n133 = case shown="17" w181 {
            tunnel: ["A" "B" "C" "D" "E" "F" "G" "H" "J" "K" "L" "M" "N" "K 5" "K 6" "K 7" "K 8" "K 9"] -> w182
            tunnel: ["String 1" "String 2" "String 3" "String 4" "String 5" "String 6" "String 7" "String 8" "String 9" "String 10" "String 11" "String 12" "String 13" "String 14" "String 15" "String 16" "String 17" "String 18"] -> w170
            frame 1, Default {
            }
            frame 2 {
            }
            frame 3 {
            }
            frame 4 {
            }
            frame 5 {
            }
            frame 6 {
            }
            frame 7 {
            }
            frame 8 {
            }
            frame 9 {
            }
            frame 10 {
            }
            frame 11 {
            }
            frame 12 {
            }
            frame 13 {
            }
            frame 14 {
            }
            frame 15 {
            }
            frame 16 {
            }
            frame 17 {
            }
            frame 18 {
            }
          }
          n134 = Add(x=65, y=w173) -> (x+y=w175:i32)
          n135 = Build Array(w175) -> (w176:i32[])
          n136 = Byte Array To String(unsigned byte array=w176) -> (string=w171:string)
          n137 = Index Array(array=w183, index=w182) -> (element=w180:string)
          n138 = Format Into String(format string="<<%s>>%s" ("Format String"), initial string=w179, w180, w170) -> (resulting string=w178:string)  [unwired: 1 in, 1 out]
          n139 = Format Into String(format string="%s%s" ("Format String"), initial string=w169, w171, w170) -> (resulting string=w168:string)  [unwired: 1 in, 1 out]
        }
        "Maths Equation Out" <- w162
        "Maths Equation Symbols" <- w160
      }
      frame "What to do next?" {
        n140 = while {
          tunnel: [w236] -> w229
          shift-left: _ -> [w236]
          shift-right: [w237] -> w230
          stop <- FALSE continue-if-true
          n141 = local read "Number of Variables"() -> (w237:i32)
        }
        n142 = Not Equal?(x=w230, y=w229) -> (x != y?=w226:bool)
        n143 = Select(t="Hide/Show", s=w226, f="Create Maths String") -> (s? t:f=w220:string)
        n144 = Select(t="End", s="OK", f=w220) -> (s? t:f=w222:string)
        n145 = Select(t="Read Maths Equation", s="Reset", f=w222) -> (s? t:f=w221:string)
      }
      frame "End" {
      }
    }
  }
  "Template Info Array Out" <- w3
